vi "Multi_Run_Prog.vi"(0 "Command filename":path, 1 "Setup mode":T9(ring)) -> ()   [LabVIEW 2014]
uses:
  Anemometry Sub Vis/Gen Trav/Traverse_cluster.ctl
  Anemometry Sub Vis/Gen Trav/Spacing.ctl
  Anemometry Sub Vis/Controls/Multi_run_mode.ctl
  Anemometry Sub Vis/Gen Trav/Route mapping/Route_Display_Mode.ctl
  Anemometry Sub Vis/Controls/User_Specific_mode.ctl
  Anemometry Sub Vis/Controls/Multi_Run_Case.ctl
  Anemometry Sub Vis/Gen Trav/Multi_Run_Status.ctl
  Anemometry Sub Vis/Controls/Tunnel_Coordinates.ctl
  Anemometry Sub Vis/Controls/Post_Process.ctl
  ADAM Client/Sub VIs/ADAM Controls/Traverse_Level_State.ctl
  ADAM Client/Sub VIs/ADAM Controls/Tunnel_speed_mode.ctl
  Anemometry Sub Vis/Controls/Overhead.ctl
  ADAM Client/Sub VIs/ADAM Controls/Remember_value_mode.ctl
  Anemometry Sub Vis/Gen Trav/Trav_mode.ctl
  Anemometry Sub Vis/Controls/Home.ctl
  ADAM Client/Sub VIs/ADAM Controls/Client_Source_Status.ctl
  ADAM Client/Sub VIs/ADAM Controls/Update_scan_value.ctl
  Anemometry Sub Vis/File/Setup_Filetype.ctl
  Anemometry Sub Vis/Globals/Meas_global.vi
  Anemometry Sub Vis/Globals/Trav_pos_global.vi
  Anemometry Sub Vis/Globals/Preference_global.vi
  Anemometry Sub Vis/Gen Trav/Route mapping/Route_mapping_global.vi
  ADAM Serial/Instrument drivers/Traverses/~subVIs/DriveConfigGlobal.vi
  Anemometry Sub Vis/Globals/Extra_Commands_Global.vi
panel:
  out "Last Row Run":i32
  in  "Stop after Repeats":bool
  in  "Jump Bad Positions":bool
  in  "Work in Tunnel Coordinates?":T1
  out "Current Overhead Factor":dbl format="%.3f"
  out "Estimated Completion time":string
  out "Max Tunnel Speed":dbl format="%.2f"
  out "Pause message":string
  in  "Pause":bool
  out "Non Starter":bool
  out "No of Rows":i32
  out "Status":T2
  in  "Synchronization Start No":i32=1 min=1 max=100
  out "Multi Run Case":T3
  out "Simulate/Run":T4
  in  "Display Mode":T5=enum."Display View on Crash"
  in  "stop":bool
  out "Currently on Row":i32
  in  "Table":T6[](array[typedef]) {"Row Duration (mins)" format="%#.1f"; "Row No" min=0; "Trace Gas Concentration (%)" min=0.0 format="%#.2f"; "Emission Rate (l/min)" format="%#.2f"; "Tunnel Speed" format="%#.2f"; "Start X" format="%#.2f"; "Start Y" format="%#.2f"; "Start Z" format="%#.2f"; "End X" format="%#.2f"; "End Y" format="%#.2f"; "End Z" format="%#.2f"; "Averaging time (min)" min=0.0 format="%#.2f"}
  # "X           Y            Z"
  # "Start"
  # "End"
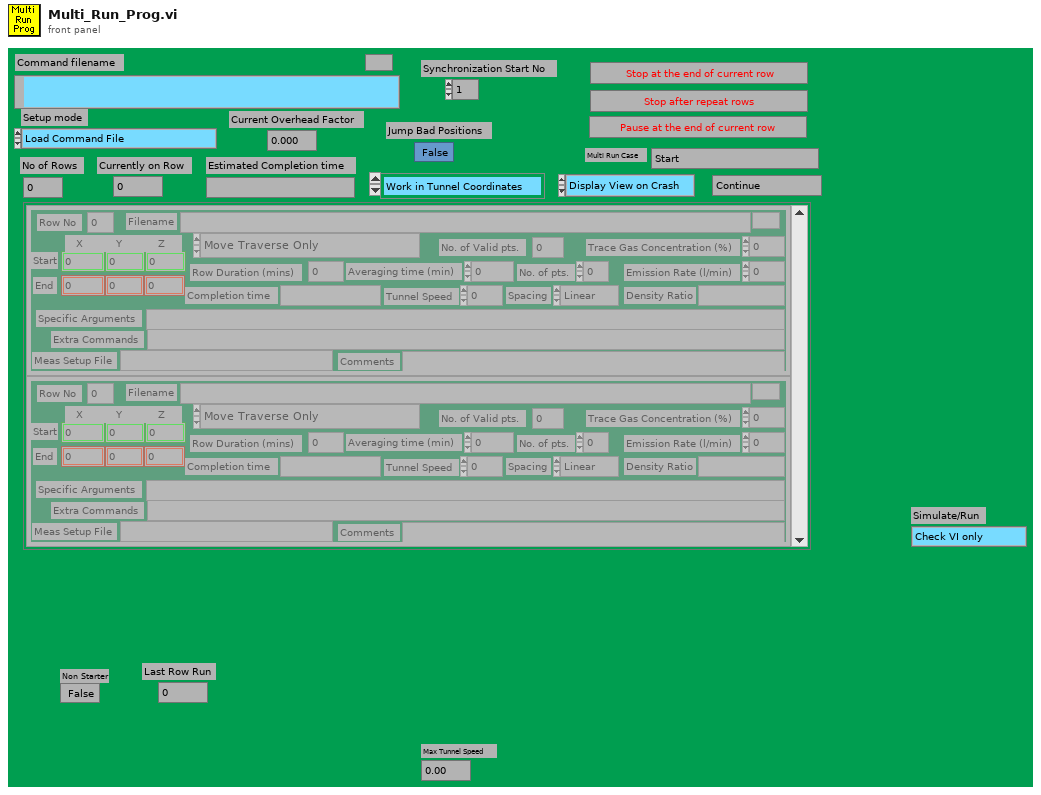
[diagram p1: front panel]
types:
  T1 = typedef "Tunnel_Coordinates.ctl" = enum16{"Work in Tunnel Coordinates", "Work in Model Coordinates"}
  T2 = typedef "Multi_Run_Status.ctl" = enum16{"Continue", "Jump to Next Point", "Jump to Next Row", "Jump To Fall Back", "Terminate Run"}
  T3 = typedef "Multi_Run_Case.ctl" = enum16{"Start", "Load Setup From File", "Has file been edited in Excel?", "Check Max Tunnel Speed", "Pre Check Row", "Check Rows", "Remove blank end rows", "Do results files already exist?", "FFID Bkgnd Measurements?", "First Save Setup file", "Setup Route checking", "Initialise Measurement Prog", "Input Current Position", "Experimental setup control", "Check source flowrates", "Setup for running mode", "Skip Blank Rows", "Which row to execute next", "Evaluate IF Statement", "Perform Measurement Setup", "Set Measurement Conditions", "Execute Row", "Calculate Row TIme", "Update time estimate", "Pause Multi Run Program", "Do Another Row?", "Find Next Fall Back Row", "Shut down source etc", "Email results to users", "Save run efficiency", "Remove Skipped Commands", "Show jumped positions", "Save Setup to File", "End"}
  T4 = typedef "User_Specific_mode.ctl" = enum16{"Check VI only", "Run VI"}
  T5 = typedef "Route_Display_Mode.ctl" = enum16{"Display View Always", "Display View on Crash"}
  T6 = typedef "Traverse_cluster.ctl" = cluster{"Start X":dbl, "Start Y":dbl, "Start Z":dbl, "End X":dbl, "End Y":dbl, "End Z":dbl, "No. of pts.":i32, "Spacing":T7, "Filename":path, "Tunnel Speed":dbl, "Averaging time (min)":dbl, "Extra Commands":string, "Specific Arguments":string, "Emission Rate (l/min)":dbl, "Trace Gas Concentration (%)":dbl, "Density Ratio":string, "Comments":string, "Row No":i32, "Row Type Selector":T8, "Completion time":string, "Row Duration (mins)":dbl, "No. of Valid pts.":i32, "Meas Setup File":string}
  T7 = typedef "Spacing.ctl" = enum16{"Linear", "Log", "Gauss", "Specified", "N/A"}
  T8 = typedef "Multi_run_mode.ctl" = enum16{"Move Traverse Only", "Set Tunnel Speed Only", "Set Source Only", "Set Measurement Conditions", "Single Measurement", "Vertical Profile", "Lateral Profile", "Longitudinal Profile", "Explore Volume", "Multi-Axis Profile", "Auto Calibrate", "Meas Fast FID Bkgnd", "Check Beam Power", "Scanning Valve Measurement", "Run VI Named:", "Set ADAM Ch", "Wait (minutes)", "Send Message", "Synchronize With:", "Fall Back to this Row", "Turn Off Row Repeating", "Blank Row", "Traverse 3D Volume"}
  T9 = enum16{"Load Command File", "Save Command File", "Check Multi Run Prog", "Check Multi Run Prog With Live Moves", "Run Multi Run Prog"}
  T10 = typedef "Post_Process.ctl" = enum16{"Take New Data", "Post Process Raw Data File"}
  T11 = typedef "Traverse_Level_State.ctl" = enum16{"Running", "Complete"}
  T12 = enum32{"existing file", "new file", "new or existing file", "existing dir", "new dir", "new or existing dir", "existing file (use LLBs)", "new file (use LLBs)", "new or existing file (use LLBs)", "new or existing file or directory (use LLBs)"}
  T13 = typedef "Tunnel_speed_mode.ctl" = enum16{"Set Speed", "Set Speed then wait", "Is tunnel speed allowable?"}
  T14 = enum16{"All Channel Names", "Valid Channel Names"}
  T15 = typedef "Overhead.ctl" = enum16{"Update total times", "Read Current Overhead", "Re Scale totals to 3 hrs", "Initialise totals to 3hr"}
  T16 = typedef "Remember_value_mode.ctl" = enum16{"Read only", "Read and Write"}
  T17 = typedef "Home.ctl" = enum16{"Don't Home", "Home  +X", "Home  -X", "Home  +Y", "Home  -Y", "Home  +Z", "Home  -Z"}
  T18 = typedef "Trav_mode.ctl" = enum16{"Move traverse", "Read traverse position", "Teach Position"}
  T19 = typedef "Client_Source_Status.ctl" = enum16{"Not Using", "Using", "Must Have"}
  T20 = typedef "Update_scan_value.ctl" = cluster{"Channel Name":string, "New Value":dbl}
  T21 = typedef "Setup_Filetype.ctl" = enum16{"Measurement Setups", "Calibration Setups", "General", "Results File Plotter Setups", "Speed Calib Tweaks"}
  T22 = typedef "AxisConfigCluster.ctl" = cluster{"Channel Properties":T23, "Static Drive Configuration":T24}
  T23 = typedef "DriveProperties.ctl" = cluster{"Channel Name":string, "Vel. Default":dbl, "Acc. Default":dbl, "Vel. Max":dbl, "Vel. Min":dbl, "Acc. Max":dbl, "Acc. Min":dbl, "Pulses/unit":dbl, "Address":u8, "Pulse Offset":i32, "Pos Tolerance":dbl, "Pulses/rev":dbl, "Backlash/Eng units":dbl, "Current Pos":dbl, "Ch Status":enum16{"Active", "Offline", "Simulate"}, "Port Name":string, "Axis Transform mode":string, "Metadata Ch Name":string, "Type":string}
  T24 = typedef "DriveStaticConfig.ctl" = cluster{"Correction Gain % (CG)":u16, "Dead Band (DB)":i32, "Dead Band Window (DW)":i32, "Encoder Resolution (ER)":i32, "Step Mode  (FSB)":u16, "Position Maintenance (FSC)":u16, "Stop on Stall (FSD)":u16, "Activate OP1 on stall (FSE)":u16, "Stop on Trigger 3 (FSF)":u16, "OP2 in Deadband (FSG)":u16, "Stall Detect (FSH)":u16, "Limit Disable (LD)":u16, "Motor Resolution (MR)":enum16{"200", "400", "1000", "2000", "4000", "5000", "10000", "12800", "18000", "20000", "21600", "25000", "25400", "25600", "36000", "50000", "278528", "425984", "507904", "614400", "655360", "819200", "1024000"}, "Limit Switch Sense (OSA)":u16, "Home Position (OSB)":u16, "Home Switch Sense (OSC)":u16, "Encoder Z for Home (OSD)":u16, "Reference edge of Home (OSH)":u16, "RS232 Echo Control (SSA)":u16, "Buffer at Limit (SSG)":u16, "Buffer at Stop (SSH)":u16, "Indexer Mode  (FSA)":u16, "Type":string, "ConfigString":string, "De Power Motor":enum16{"TRUE", "FALSE"}}
  T25 = typedef "Status_Cluster.ctl" = cluster{"Status":T2, "Error Type":string, "Error Description":string}
  T26 = typedef "Server_Comms.ctl" = enum16{"Server Link Healthy", "Do Not Link To Server"}
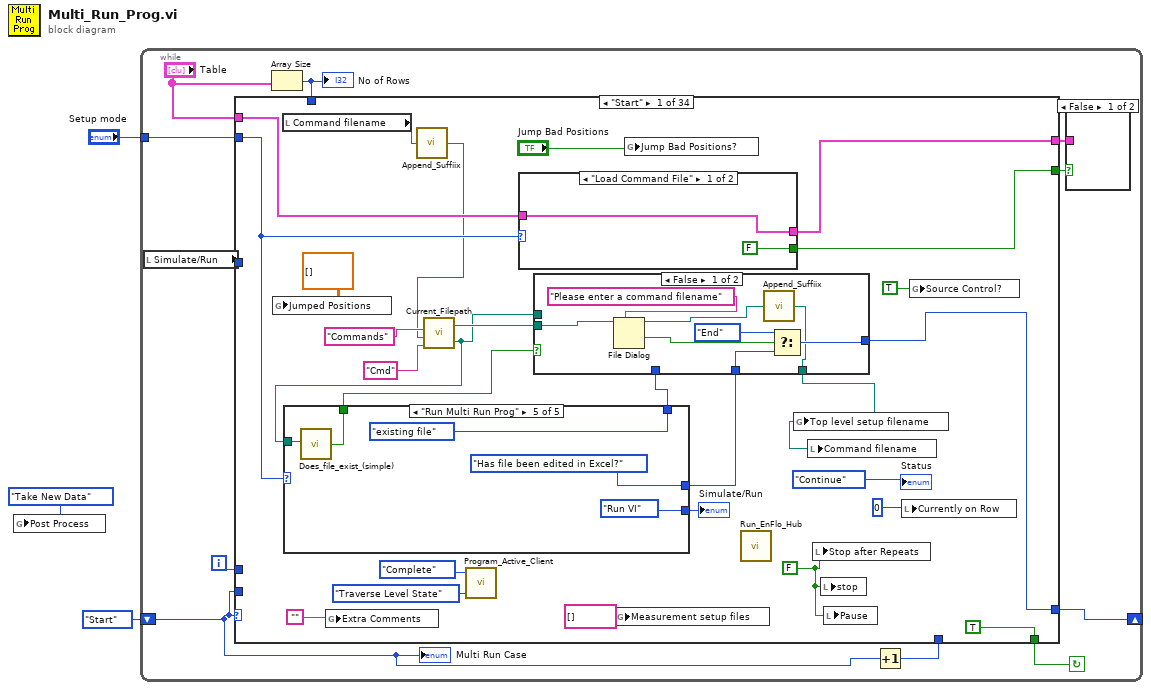
[diagram p0: block diagram]
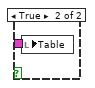
[diagram p2: hidden frame]
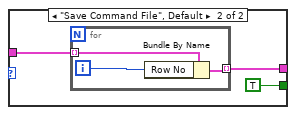
[diagram p3: hidden frame]
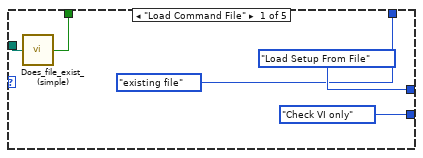
[diagram p5: hidden frame]
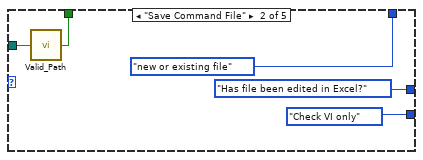
[diagram p6: hidden frame]
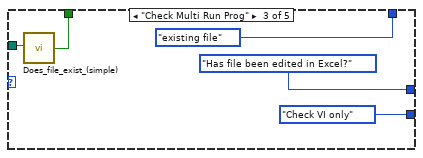
[diagram p7: hidden frame]
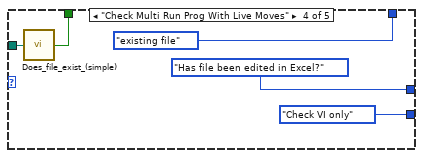
[diagram p8: hidden frame]
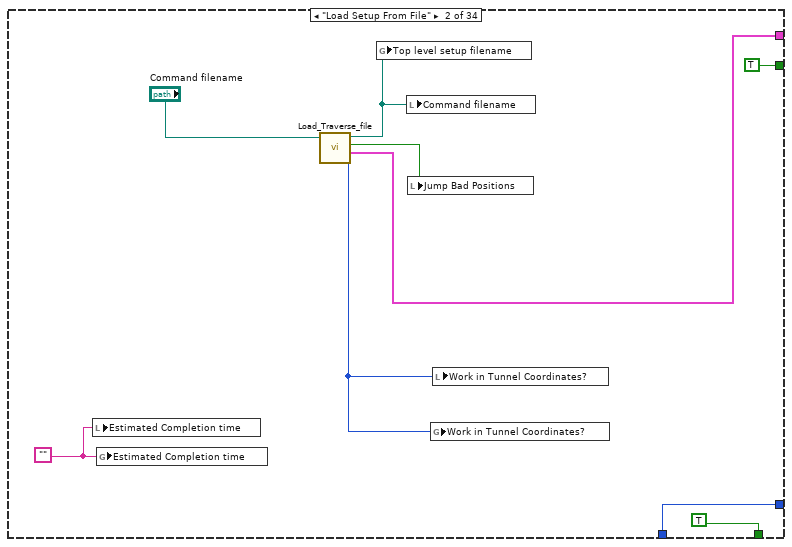
[diagram p9: hidden frame]
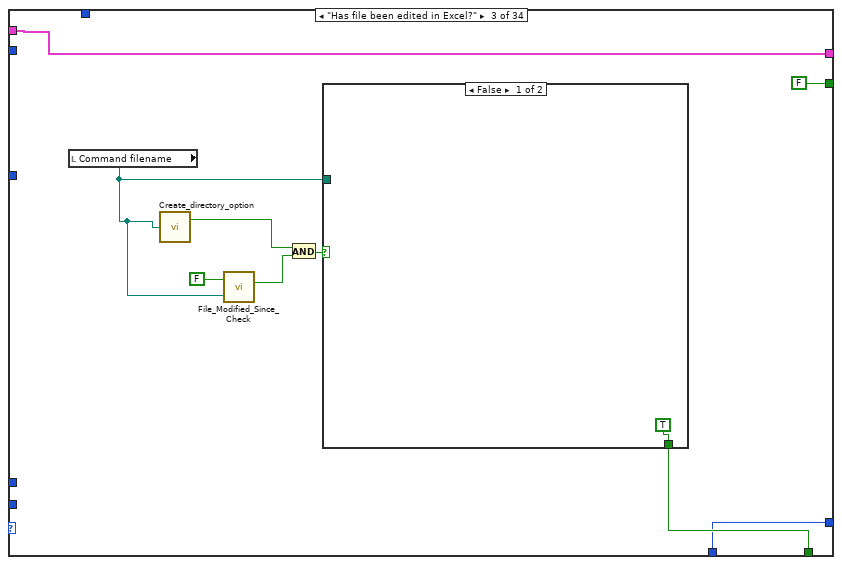
[diagram p10: hidden frame]
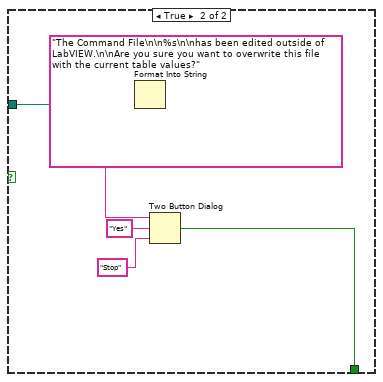
[diagram p11: hidden frame]
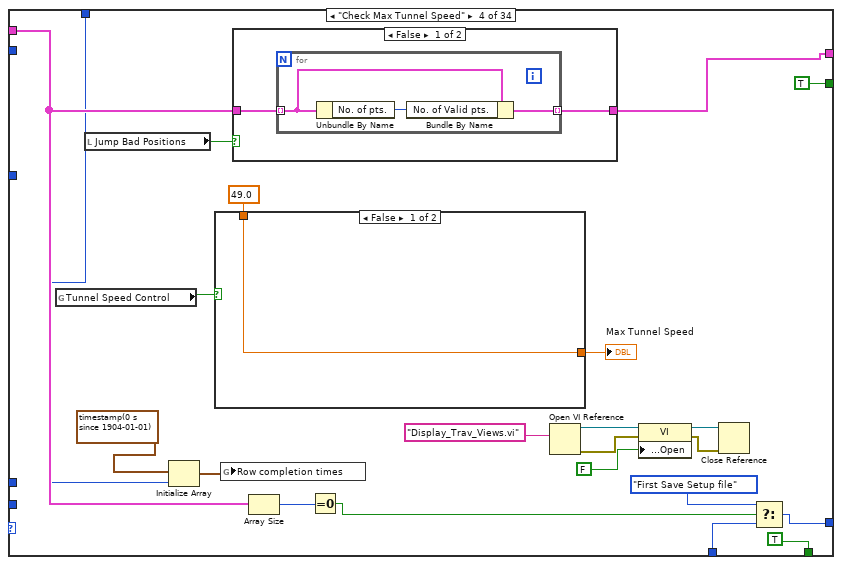
[diagram p12: hidden frame]
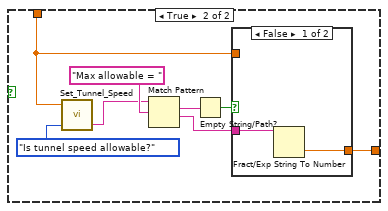
[diagram p14: hidden frame]
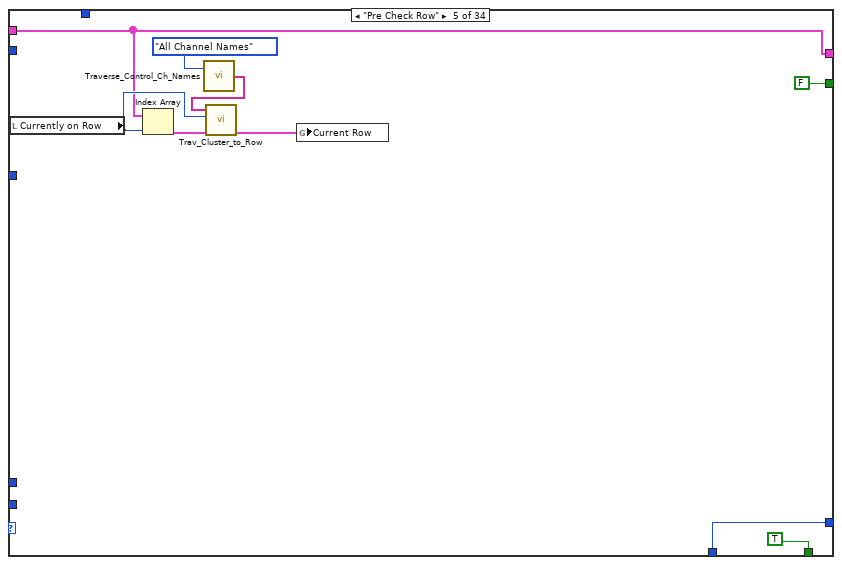
[diagram p16: hidden frame]
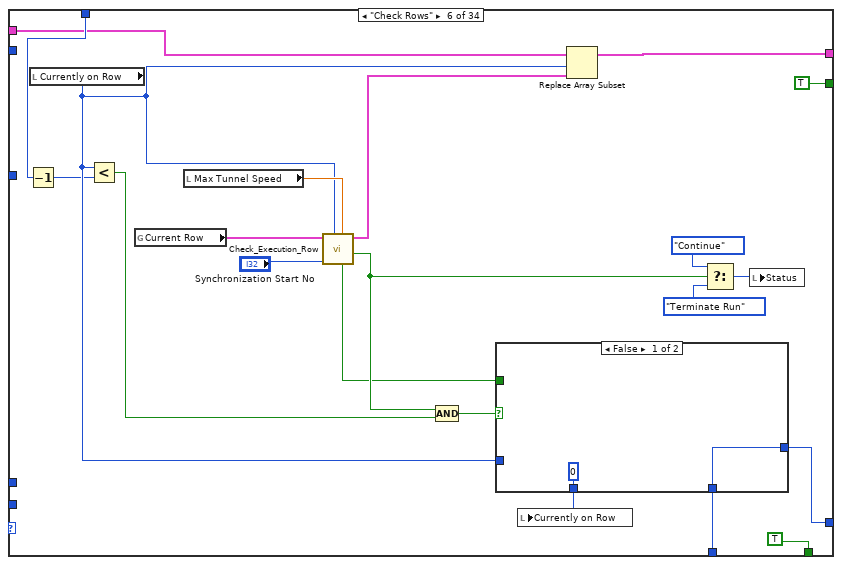
[diagram p17: hidden frame]
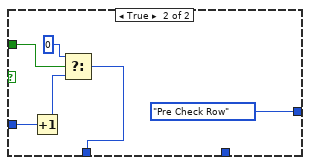
[diagram p18: hidden frame]
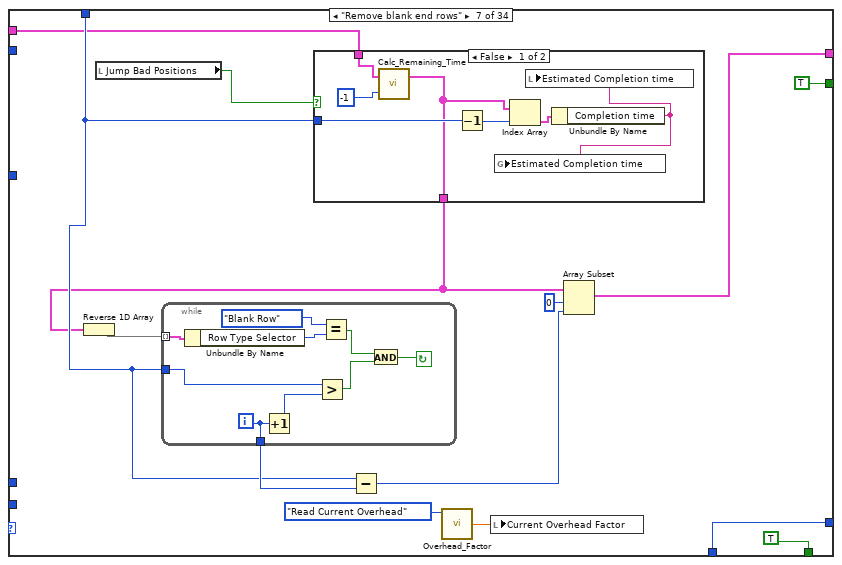
[diagram p19: hidden frame]
diagram:
  n1 = global write "Meas_global.vi" "Post Process"(Post_Process."Take New Data" ("Post Process")) -> ()
  n2 = while {
    shift-left: Multi_Run_Case."Start" ("Multi Run Case") -> [w10]
    shift-right: [w6] -> _
    tunnel: "Setup mode" -> [w13]
    i -> [w11]
    stop <- w14 continue-if-true
    n3 = local read "Simulate/Run"() -> (w7:T4)
    n4 = Array Size(array="Table") -> (size(s)=w5:i32)
    "No of Rows" <- w5
    n5 = Increment(x=w10) -> (x+1=w12:T3)
    n6 = case shown="\"Start\"" w10 {
      tunnel: [TRUE TRUE w98 TRUE TRUE TRUE TRUE TRUE TRUE TRUE TRUE ("Continue?") TRUE ("Continue?") TRUE TRUE TRUE w518 TRUE ("Continue?") TRUE ("Continue?") TRUE TRUE ("Continue?") TRUE TRUE TRUE TRUE TRUE TRUE TRUE TRUE TRUE TRUE TRUE TRUE TRUE FALSE] -> w14
      tunnel: w13 -> [w28 _ _ _ _ _ _ _ _ w406 _ _ _ _ _ _ _ _ _ _ _ _ _ _ _ _ _ _ _ _ _ _ w1268 _]
      tunnel: "Table" -> [w40 _ w95 w125 w153 w165 w190 w221 w379 w408 w430 w484 w489 w495 w505 w521 w596 w640 w756 w807 w819 w912 w948 w980 w1023 w1069 w1117 w1145 w1165 w1212 w1217 w1226 w1289 w1353]
      tunnel: w7 -> [_ _ _ _ _ _ _ w220 _ _ _ _ _ w499 w504 w520 _ w638 w753 w804 w817 w911 w946 w977 _ w1078 _ _ _ _ _ _ w1279 _]
      tunnel: w10 -> [_ _ _ _ _ _ _ _ _ _ _ _ _ _ _ _ _ _ _ _ _ _ _ _ _ _ _ _ _ _ _ _ _ _]
      tunnel: w12 -> [_ w91 w97 w123 w157 w167 w201 w225 w374 w405 w434 w482 w490 w494 w510 w523 w598 w636 w761 w808 w826 w909 w938 w982 w1026 _ _ w1131 w1167 w1214 w1220 w1234 w1287 w1352]
      tunnel: w11 -> [_ _ _ _ _ _ _ _ _ _ _ _ _ _ _ _ _ _ _ _ _ _ _ _ w1024 _ _ _ _ _ _ _ _ _]
      tunnel: [w38 w91 w97 w122 w157 w166 w201 w225 w374 w401 w434 w481 w490 w494 w507 w523 w598 w637 w760 w808 w827 w909 w938 w982 w1027 w1061 w1114 w1140 w1167 w1214 w1220 w1234 w1287 w1352] -> w6
      tunnel: [w27 TRUE FALSE ("Rows Added ?") TRUE ("Rows Added ?") FALSE TRUE TRUE FALSE FALSE TRUE FALSE FALSE FALSE FALSE FALSE TRUE FALSE ("Rows Added ?") FALSE ("Rows Added ?") FALSE FALSE ("Rows Added ?") FALSE FALSE FALSE TRUE ("Rows Added ?") FALSE FALSE FALSE FALSE FALSE FALSE TRUE TRUE TRUE FALSE] -> w8
      tunnel: w5 -> [_ _ _ w117 _ w171 w192 _ _ _ _ _ _ _ _ _ w599 w639 _ _ _ _ _ w976 _ w1064 _ _ _ _ _ _ _ _]
      tunnel: [w39 w92 w95 w127 w153 w174 w196 w221 w379 w409 w430 w484 w489 w495 w505 w519 w596 w641 w756 w807 w819 w912 w948 w979 w1023 w1069 w1117 w1145 w1165 w1212 w1216 w1226 w1288 w1353] -> w4
      frame "Start" {
        w25 = FALSE ("Measurment setup Found?")
        n7 = global write "Trav_pos_global.vi" "Jumped Positions"(dbl[][] [] ("Jumped Positions")) -> ()
        n8 = local read "Command filename"() -> (w30:path)
        n9 = global write "Meas_global.vi" "Extra Comments"("") -> ()
        n10 = call "Append_Suffiix.vi"("Results file"=w30) -> ("appended path"=w20:path)
        n11 = call "Current_Filepath.vi"("Short_Name"="Cmd" ("Data Type"), "Filename in"=w20, "Data Type"="Commands") -> ("Filename Out"=w17:path, "Directory"=w19:path)  [unwired: 1 in]
        n12 = case shown="\"Run Multi Run Prog\"" w28 {
          tunnel: [User_Specific_mode."Check VI only" ("Simulate/Run") User_Specific_mode."Check VI only" ("Simulate/Run") User_Specific_mode."Check VI only" ("Simulate/Run") User_Specific_mode."Check VI only" ("Simulate/Run") User_Specific_mode."Run VI" ("Simulate/Run")] -> w41
          tunnel: [Multi_Run_Case."Load Setup From File" ("Multi Run Case") Multi_Run_Case."Has file been edited in Excel?" ("Multi Run Case") Multi_Run_Case."Has file been edited in Excel?" ("Multi Run Case") Multi_Run_Case."Has file been edited in Excel?" ("Multi Run Case") Multi_Run_Case."Has file been edited in Excel?" ("Multi Run Case")] -> w37
          tunnel: [T12."existing file" ("select mode (2)") T12."new or existing file" ("select mode (2)") T12."existing file" ("select mode (2)") T12."existing file" ("select mode (2)") T12."existing file" ("select mode (2)")] -> w26
          tunnel: w17 -> [w62 w67 w71 w77 w82]
          tunnel: [w61 w66 w72 w76 w81] -> w16
          frame "Load Command File" {
            n13 = call "Does_file_exist_(simple).vi"("Pathname"=w62) -> ("exists?"=w61:bool)
          }
          frame "Save Command File" {
            n14 = call "Valid_Path.vi"("Filename"=w67) -> ("Valid Path?"=w66:bool)
          }
          frame "Check Multi Run Prog" {
            n15 = call "Does_file_exist_(simple).vi"("Pathname"=w71) -> ("exists?"=w72:bool)
          }
          frame "Check Multi Run Prog With Live Moves" {
            n16 = call "Does_file_exist_(simple).vi"("Pathname"=w77) -> ("exists?"=w76:bool)
          }
          frame "Run Multi Run Prog" {
            n17 = call "Does_file_exist_(simple).vi"("Pathname"=w82) -> ("exists?"=w81:bool)
          }
        }
        "Simulate/Run" <- w41
        n18 = call "Program_Active_Client.vi"("Mode"=enum16{"Program Active", "Traverse Level State"}."Traverse Level State", "Traverse level State"=Traverse_Level_State."Complete") -> ()  [unwired: 1 in, 3 out]
        n19 = case shown="\"Load Command File\"" w28 {
          tunnel: w40 -> [w44 w47]
          tunnel: [w44 w46] -> w39
          tunnel: [FALSE TRUE] -> w27
          frame "Load Command File" {
          }
          frame "Save Command File", Default {
            n20 = for {
              tunnel: w47 -> [w50] mode=indexing
              tunnel: [w49] -> w46 mode=indexing
              i -> [w48]
              n21 = Bundle By Name(cluster=w50, "Row No"=w48) -> (w49:T6)
            }
          }
        }
        n22 = case shown="False" w16 {
          tunnel: [w56 w60] -> w38
          tunnel: w37 -> [w57 w60]
          tunnel: w17 -> [_ w59]
          tunnel: [w55 w59] -> w29
          tunnel: w26 -> [_ _]
          tunnel: w19 -> [w51 _]
          frame False {
            n23 = File Dialog(7:"Please enter a command filename" ("prompt"), 11:w51) -> (1:w53:bool, 3:w54:path)  [unwired: 1 in, 6 out]
            n24 = call "Append_Suffiix.vi"("Results file"=w54) -> ("appended path"=w55:path)
            n25 = Select(t=Multi_Run_Case."End" ("Multi Run Case"), s=w53, f=w57) -> (s? t:f=w56:T3)
          }
          frame True {
          }
        }
        n26 = global write "Trav_pos_global.vi" "Measurement setup files"(string[] [] ("Measurement setup files")) -> ()
        n27 = global write "Trav_pos_global.vi" "Jump Bad Positions?"("Jump Bad Positions") -> ()
        n28 = call "Run_EnFlo_Hub.vi"() -> ()  [unwired: 8 out]
        n29 = global write "Trav_pos_global.vi" "Top level setup filename"(w29) -> ()
        n30 = local write "Command filename"(w29) -> ()
        n31 = local write "Stop after Repeats"(w25) -> ()
        n32 = local write "stop"(w25) -> ()
        n33 = local write "Pause"(w25) -> ()
        n34 = local write "Currently on Row"(0 ("Currently on Row")) -> ()
        n35 = global write "Trav_pos_global.vi" "Source Control?"(TRUE ("Source Control?")) -> ()
        "Status" <- Multi_Run_Status."Continue" ("Status")
      }
      frame "Load Setup From File" {
        w87 = ""
        n36 = local write "Estimated Completion time"(w87) -> ()
        n37 = global write "Trav_pos_global.vi" "Estimated Completion time"(w87) -> ()
        n38 = call "Load_Traverse_file.vi"("Setup filename"="Command filename") -> ("Setup filename Out"=w89:path, "Jump Bad Positions"=w86:bool, "Table"=w92:T6[], "Work in Tunnel Coordinates?"=w88:T1)  [unwired: 2 out]
        n39 = global write "Trav_pos_global.vi" "Top level setup filename"(w89) -> ()
        n40 = local write "Command filename"(w89) -> ()
        n41 = local write "Jump Bad Positions"(w86) -> ()
        n42 = global write "Trav_pos_global.vi" "Work in Tunnel Coordinates?"(w88) -> ()
        n43 = local write "Work in Tunnel Coordinates?"(w88) -> ()
      }
      frame "Has file been edited in Excel?" {
        n44 = local read "Command filename"() -> (w99:path)
        n45 = call "Create_directory_option.vi"("Filename"=w99) -> ("Path is to existing File"=w102:bool)  [unwired: 1 out]
        n46 = call "File_Modified_Since_Check.vi"("Pathname"=w99, "Just Modified?"=FALSE) -> ("Modified?"=w101:bool)
        n47 = And(x=w102, y=w101) -> (x .and. y?=w103:bool)
        n48 = case shown="False" w103 {
          tunnel: w99 -> [_ w110]
          tunnel: [TRUE ("T button?") w105] -> w98
          frame False {
          }
          frame True {
            n49 = Format Into String(format string="The Command File\n\n%s\n\nhas been edited outside of LabVIEW.\n\nAre you sure you want to overwrite this file  with the current table values?" ("Format String"), w110) -> (resulting string=w108:string)  [unwired: 2 in, 1 out]
            n50 = Two Button Dialog(message=w108, 1:"Stop" ("F button name (\"Cancel\")"), 2:"Yes" ("T button name (\"OK\")")) -> (T button?=w105:bool)
          }
        }
      }
      frame "Check Max Tunnel Speed" {
        n51 = global read "Preference_global.vi" "Tunnel Speed Control"() -> (w128:bool)
        n52 = local read "Jump Bad Positions"() -> (w126:bool)
        n53 = Initialize Array(timestamp(0 s since 1904-01-01) ("seconds since 1Jan1904"), w117) -> (w118:timestamp[])
        n54 = case shown="False" w128 {
          tunnel: 49.0 ("Tunnel Velocity m/s") -> [w139 w140]
          tunnel: [w139 w142] -> w130
          frame False {
          }
          frame True {
            n55 = call "Set_Tunnel_Speed.vi"("Mode"=Tunnel_speed_mode."Is tunnel speed allowable?", "Tunnel Velocity m/s"=w140) -> ("Error String"=w145:string)  [unwired: 1 in, 2 out]
            n56 = Match Pattern(string=w145, regular expression="Max allowable = ") -> (match substring=w144:string, after substring=w141:string)  [unwired: 3 out]
            n57 = Empty String/Path?(string/path=w144) -> (empty?=w143:bool)
            n58 = case shown="False" w143 {
              tunnel: [w148 w150] -> w142
              tunnel: w140 -> [_ w150]
              tunnel: w141 -> [w149 _]
              frame False {
                n59 = Fract/Exp String To Number(string=w149) -> (number=w148:dbl)  [unwired: 4 out]
              }
              frame True {
              }
            }
          }
        }
        "Max Tunnel Speed" <- w130
        n60 = global write "Trav_pos_global.vi" "Row completion times"(w118) -> ()
        n61 = case shown="False" w126 {
          tunnel: w125 -> [w134 w138]
          tunnel: [w133 w138] -> w127
          frame False {
            n62 = for {
              tunnel: w134 -> [w136] mode=indexing
              tunnel: [w135] -> w133 mode=indexing
              n63 = Unbundle By Name(w136) -> ("No. of pts."=w137:i32)
              n64 = Bundle By Name(cluster=w136, "No. of Valid pts."=w137) -> (w135:T6)
            }
          }
          frame True {
          }
        }
        n65 = Array Size(array=w125) -> (size(s)=w124:i32)
        n66 = Equal To 0?(x=w124) -> (x = 0?=w121:bool)
        n67 = Open VI Reference(vi path="Display_Trav_Views.vi" ("VI path")) -> (vi reference=w116:refnum<vi>, error out=w115:errorcluster)  [unwired: 1 in, 4 out]
        n68 = property class="VI"(reference=w116, error in=w115, "Front Panel Window:Open"=FALSE) -> (reference out=w113:refnum<vi>, error out=w112:errorcluster)
        n69 = Close Reference(reference=w113, error in (no error)=w112) -> ()  [unwired: 1 out]
        n70 = Select(t=Multi_Run_Case."First Save Setup file" ("Multi Run Case"), s=w121, f=w123) -> (s? t:f=w122:T3)
      }
      frame "Pre Check Row" {
        n71 = local read "Currently on Row"() -> (w154:i32)
        n72 = Index Array(array=w153, index=w154) -> (element=w155:T6)
        n73 = call "Traverse_Control_Ch_Names.vi"("Mode"=T14."All Channel Names") -> ("Channel names"=w151:string[])  [unwired: 1 in]
        n74 = call "Trav_Cluster_to_Row.vi"("Traverse line in"=w155, "Row Number"=w154, "Channel names"=w151) -> ("Traverse line Out"=w156:T6)  [unwired: 4 out]
        n75 = global write "Trav_pos_global.vi" "Current Row"(w156) -> ()
      }
      frame "Check Rows" {
        n76 = Decrement(x=w171) -> (x-1=w162:i32)
        n77 = local read "Currently on Row"() -> (w163:i32)
        n78 = Less?(x=w163, y=w162) -> (x < y?=w170:bool)
        n79 = global read "Trav_pos_global.vi" "Current Row"() -> (w160:T6)
        n80 = local read "Max Tunnel Speed"() -> (w173:dbl)
        n81 = call "Check_Execution_Row.vi"("Execution Row"=w160, "Synchronization Start No"="Synchronization Start No", "Row Index"=w163, "Max Tunnel Speed"=w173) -> ("Editted Row"=w161:bool, "Execution Row Out"=w164:T6, "Continue?"=w172:bool)  [unwired: 1 in, 3 out]
        n82 = Compound Arithmetic op=AND(w172, w170) -> (w169:bool)
        n83 = case shown="False" w169 {
          tunnel: [0 w184] -> w168
          tunnel: w163 -> [_ w188]
          tunnel: w167 -> [w182 _]
          tunnel: [w182 Multi_Run_Case."Pre Check Row" ("Multi Run Case")] -> w166
          tunnel: w161 -> [_ w186]
          frame False {
          }
          frame True {
            n84 = Increment(x=w188) -> (x+1=w185:i32)
            n85 = Select(t=0, s=w186, f=w185) -> (s? t:f=w184:i32)
          }
        }
        n86 = local write "Currently on Row"(w168) -> ()
        n87 = Replace Array Subset(array=w165, new element=w164, index=w163) -> (w174:T6[])
        n88 = Select(t=Multi_Run_Status."Continue" ("Status"), s=w172, f=Multi_Run_Status."Terminate Run" ("Status")) -> (s? t:f=w178:T2)
        n89 = local write "Status"(w178) -> ()
      }
      frame "Remove blank end rows" {
        n90 = local read "Jump Bad Positions"() -> (w189:bool)
        n91 = case shown="False" w189 {
          tunnel: w192 -> [w207 _]
          tunnel: w190 -> [w206 w210]
          tunnel: [w204 w210] -> w191
          frame False {
            n92 = call "Calc_Remaining_Time.vi"("Currently on Row"=-1 ("Start Index"), "Table In"=w206) -> ("Table Out"=w204:T6[])  [unwired: 1 out]
            n93 = Decrement(x=w207) -> (x-1=w209:i32)
            n94 = Index Array(array=w204, index=w209) -> (element=w208:T6)
            n95 = Unbundle By Name(w208) -> ("Completion time"=w203:string)
            n96 = global write "Trav_pos_global.vi" "Estimated Completion time"(w203) -> ()
            n97 = local write "Estimated Completion time"(w203) -> ()
          }
          frame True {
          }
        }
        n98 = Reverse 1D Array(array=w191) -> (reversed array=w200:T6[])
        n99 = while {
          tunnel: [w211] -> w198
          tunnel: w192 -> [w215]
          tunnel: w200 -> [w219] mode=indexing
          i -> [w211]
          stop <- w212 continue-if-true
          n100 = Unbundle By Name(w219) -> ("Row Type Selector"=w217:T8)
          n101 = Increment(x=w211) -> (x+1=w216:i32)
          n102 = Greater?(x=w215, y=w216) -> (0:w214:bool)
          n103 = Equal?(x=Multi_run_mode."Blank Row" ("Row Type Selector"), y=w217) -> (x = y?=w213:bool)
          n104 = And(x=w213, y=w214) -> (x .and. y?=w212:bool)
        }
        n105 = Subtract(x=w192, y=w198) -> (x-y=w197:i32)
        n106 = call "Overhead_Factor.vi"("Mode"=Overhead."Read Current Overhead") -> ("Current Overhead Factor"=w193:dbl)  [unwired: 3 in]
        n107 = local write "Current Overhead Factor"(w193) -> ()
        n108 = Array Subset(array=w191, index=0 ("Array Index"), length=w197) -> (w196:T6[])
      }
      frame "Do results files already exist?" {
        n109 = for {
          tunnel: w221 -> [w237] mode=indexing
          tunnel: [w235] -> w227 mode=indexing
          shift-right: [w231] -> _
          shift-left: path[] [] -> [w232]
          tunnel: w220 -> [w229]
          n110 = Unbundle By Name(w237) -> ("Specific Arguments"=w228:string, "Emission Rate (l/min)"=w236:dbl, "Row Type Selector"=w234:T8, "Filename"=w233:path)
          n111 = while {
            shift-left: w232 -> [w245]
            shift-right: [w244] -> w231
            tunnel: w233 -> [w246]
            tunnel: w234 -> [w250]
            shift-left: 0 -> [w251]
            shift-right: [w247] -> _
            tunnel: w229 -> [w241]
            shift-right: [w240] -> _
            shift-left: _ -> [w239]
            tunnel: w228 -> [w238]
            stop <- w249 continue-if-true
            n112 = Increment(x=w251) -> (x+1=w248:i32)
            n113 = case shown="0, Default" w251 {
              tunnel: w250 -> [w260 _ _ _ _ _ _ _ _ _ _ _]
              tunnel: [w255 w280 w285 w292 w297 TRUE ("exists?") TRUE ("exists?") FALSE ("exists?") FALSE ("exists?") TRUE ("true") w354 w367] -> w249
              tunnel: w248 -> [w262 w283 w288 w291 w298 w303 w314 w325 w336 w340 w352 _]
              tunnel: [w262 w283 w288 w291 w298 w301 w313 w325 w336 w341 w352 w366] -> w247
              tunnel: [w261 w282 w287 w290 w295 w311 w322 w327 w329 w338 w356 w372] -> w244
              tunnel: w245 -> [w261 w282 w287 w290 w296 w311 w322 w327 w329 w338 w356 w372]
              tunnel: w246 -> [w254 _ _ _ _ _ _ _ _ _ _ _]
              tunnel: 7 -> [_ _ _ _ _ _ _ _ _ w339 _ w366]
              tunnel: 9 -> [_ _ _ _ _ w302 _ _ _ _ _ _]
              tunnel: w241 -> [_ _ _ _ _ _ _ _ _ _ w355 _]
              tunnel: [w253 w279 w284 w289 w294 w299 w312 w323 w328 w337 w353 w365] -> w240
              tunnel: w239 -> [_ w279 w284 w289 w294 w299 w312 w323 w328 w337 w353 w365]
              tunnel: w238 -> [w252 _ _ _ _ _ _ _ _ _ _ _]
              frame 0, Default {
                n114 = case shown="\"Send Message\"" w260 {
                  tunnel: [TRUE w270 FALSE FALSE] -> w257
                  tunnel: w254 -> [w263 w269 w275 w277]
                  tunnel: w252 -> [_ w267 _ _]
                  tunnel: [w263 w269 w275 w277] -> w253
                  frame "Move Traverse Only", Default {
                  }
                  frame "Run VI Named:" {
                    n115 = Match Pattern(string=w267, regular expression=";") -> (before substring=w266:string)  [unwired: 4 out]
                    n116 = call <vilib>:"Trim Whitespace.vi"("string"=w266) -> ("trimmed string"=w265:string)  [unwired: 1 in]
                    n117 = Equal?(x=w265, y="Pressure_Tapped_Cube.vi") -> (x = y?=w271:bool)
                    n118 = Equal?(x=w265, y="Take_Data_on_the_Move.vi") -> (x = y?=w272:bool)
                    n119 = Or(x=w271, y=w272) -> (x .or. y?=w270:bool)
                  }
                  frame "Auto Calibrate" {
                  }
                  frame "Send Message" {
                  }
                }
                n120 = local read "Status"() -> (w258:T2)
                n121 = Not Equal?(x=Multi_Run_Status."Terminate Run" ("Status"), y=w258) -> (x != y?=w256:bool)
                n122 = And(x=w257, y=w256) -> (x .and. y?=w255:bool)
              }
              frame 1 {
                n123 = Not Equal?(x=path "", y=w279) -> (x != y?=w280:bool)
              }
              frame 2 {
                n124 = Not Equal?(x=w284, y=path "") -> (x != y?=w285:bool)
              }
              frame 3 {
                n125 = Search 1D Array(1D array=w290, element=w289) -> (index of element=w293:i32)  [unwired: 1 out]
                n126 = Less Than 0?(x=w293) -> (x < 0?=w292:bool)
              }
              frame 4 {
                n127 = Build Array (concatenate)(w296, w294) -> (w295:path[])
                n128 = call "Does_file_exist_(simple).vi"("Pathname"=w294) -> ("exists?"=w297:bool)
              }
              frame 5 {
                n129 = Path To String(path=w299) -> (string=w310:string)
                n130 = global read "Meas_global.vi" "Start Time of experiment"() -> (w305:dbl)
                n131 = Concatenate Strings(w310, "Append" ("Substring")) -> (w308:string)
                n132 = call "Remember_value.vi"("Mode"=Remember_value_mode."Read only", "Ch name"=w308) -> ("Output Value"=w306:dbl)  [unwired: 1 in]
                n133 = Not Equal?(x=w305, y=w306) -> (x != y?=w304:bool)
                n134 = Select(t=w303, s=w304, f=w302) -> (s? t:f=w301:i32)
              }
              frame 6 {
                n135 = Increment(x=w314) -> (x+1=w315:i32)
                n136 = Format Into String(format string="The results filename \"%s\" already exists.\nDo you wish to append to this file during the run?" ("Format String"), w312) -> (resulting string=w319:string)  [unwired: 2 in, 1 out]
                n137 = Two Button Dialog(message=w319, 1:"Abort Run" ("F button name (\"Cancel\")"), 2:"Append" ("T button name (\"OK\")")) -> (T button?=w316:bool)
                n138 = Select(t=w315, s=w316, f=w314) -> (s? t:f=w313:i32)
              }
              frame 7 {
                n139 = local write "Status"(Multi_Run_Status."Terminate Run" ("Status")) -> ()
              }
              frame 8 {
                n140 = Path To String(path=w328) -> (string=w335:string)
                n141 = Concatenate Strings(w335, "Append" ("Substring")) -> (w333:string)
                n142 = global read "Meas_global.vi" "Start Time of experiment"() -> (w330:dbl)
                n143 = call "Remember_value.vi"("Mode"=Remember_value_mode."Read and Write", "Input Value"=w330, "Ch name"=w333) -> ()  [unwired: 1 out]
              }
              frame 9 {
                n144 = call "Read_File_Simple.vi"("Filename"=w337) -> ("string"=w344:string)  [unwired: 2 in, 7 out]
                n145 = call "Is_it_a_Results_File.vi"("character string"=w344) -> ("Results File?"=w343:bool)  [unwired: 2 out]
                n146 = case shown="True" w343 {
                  tunnel: w337 -> [w347 _]
                  tunnel: [w345 w351] -> w341
                  tunnel: w340 -> [_ w351]
                  tunnel: w339 -> [w345 _]
                  frame False {
                    n147 = Path To String(path=w347) -> (string=w349:string)
                    n148 = Format Into String(format string="The File %s is not in the correct Results file format.\nCheck that it is tab delimited rather than excel format, or choose another file." ("Format String"), w349) -> (resulting string=w346:string)  [unwired: 2 in, 1 out]
                    n149 = One Button Dialog(message=w346, button name ("OK")="Stop") -> ()  [unwired: 1 out]
                  }
                  frame True {
                  }
                }
              }
              frame 10 {
                n150 = case shown="\"Check VI only\", Default" w355 {
                  tunnel: w353 -> [_ w364]
                  tunnel: [FALSE ("exists?") w358] -> w354
                  frame "Check VI only", Default {
                  }
                  frame "Run VI" {
                    n151 = call "Open_File_for_write.vi"("append to file? (new file:F)"=TRUE, "file path"=w364) -> ("error out"=w362:errorcluster, "refnum"=w363:refnum<file>)  [unwired: 1 in, 7 out]
                    n152 = Unbundle By Name(w362) -> ("code"=w361:i32)
                    n153 = Close File(refnum=w363, error in=w362) -> ()  [unwired: 2 out]
                    n154 = Equal?(x=10 ("code"), y=w361) -> (x = y?=w358:bool)
                  }
                }
              }
              frame 11 {
                n155 = Path To String(path=w365) -> (string=w370:string)
                n156 = Format Into String(format string="The File %s is already open in another application." ("Format String"), w370) -> (resulting string=w369:string)  [unwired: 2 in, 1 out]
                n157 = One Button Dialog(message=w369, button name ("OK")="Stop") -> (true=w367:bool)
              }
            }
          }
          n158 = Greater Than 0?(x=w236) -> (x > 0?=w235:bool)
        }
        n159 = Or Array Elements(Boolean array=w227) -> (logical OR=w223:bool)
        n160 = global write "Trav_pos_global.vi" "Source Control?"(w223) -> ()
      }
      frame "FFID Bkgnd Measurements?" {
        n161 = for {
          tunnel: w379 -> [w395] mode=indexing
          tunnel: [w383] -> w378 mode=indexing
          tunnel: [w384] -> w377 mode=indexing
          n162 = Unbundle By Name(w395) -> ("Row Type Selector"=w389:T8, "Specific Arguments"=w391:string)
          n163 = call "Get_array_values_fr_String.vi"("String Value"=w391) -> ("String array"=w392:string[])  [unwired: 1 out]
          n164 = Index Array(array=w392, index=0 ("Index")) -> (element=w388:string)
          n165 = Equal?(x=Multi_run_mode."Auto Calibrate" ("Row Type Selector"), y=w389) -> (x = y?=w385:bool)
          n166 = Equal?(x=w388, y="Concentration") -> (x = y?=w386:bool)
          n167 = Equal?(x=Multi_run_mode."Meas Fast FID Bkgnd" ("Row Type Selector"), y=w389) -> (x = y?=w383:bool)
          n168 = And(x=w385, y=w386) -> (x .and. y?=w384:bool)
        }
        n169 = Or Array Elements(Boolean array=w378) -> (logical OR=w375:bool)
        n170 = Or Array Elements(Boolean array=w377) -> (logical OR=w376:bool)
        n171 = Compound Arithmetic op=AND(invert w375, w376) -> (w373:bool)
        n172 = case shown="True" w373 {
          frame False {
          }
          frame True {
            n173 = One Button Dialog(message="This run automatically calibrates the Fast FID but does not have a Meas Fast FID Bkgnd row" ("format string")) -> ()  [unwired: 2 out]
          }
        }
      }
      frame "First Save Setup file" {
        w396 = -1 ("Currently on Row")
        n174 = case shown="\"Check Multi Run Prog\"" w406 {
          tunnel: [w413 w415 w417 Multi_Run_Case."End" ("Multi Run Case") Multi_Run_Case."End" ("Multi Run Case")] -> w400
          tunnel: w405 -> [w413 w415 w417 _ _]
          tunnel: [w414 w416 w418 w419 w421] -> w399
          frame "Run Multi Run Prog" {
            w414 = FALSE  # Live Traverse Preview?
          }
          frame "Check Multi Run Prog With Live Moves" {
            w416 = TRUE  # Live Traverse Preview?
          }
          frame "Check Multi Run Prog" {
            w418 = FALSE  # Live Traverse Preview?
          }
          frame "Load Command File" {
            w419 = FALSE  # Live Traverse Preview?
          }
          frame "Save Command File" {
            w421 = FALSE  # Live Traverse Preview?
          }
        }
        n175 = local read "Command filename"() -> (w407:path)
        n176 = global write "Trav_pos_global.vi" "Work in Tunnel Coordinates?"("Work in Tunnel Coordinates?") -> ()
        n177 = local write "Currently on Row"(w396) -> ()
        n178 = local write "Last Row Run"(w396) -> ()
        n179 = local read "Jump Bad Positions"() -> (w397:bool)
        n180 = call "Save_Trav_setup.vi"("Work in Tunnel Coordinates?"="Work in Tunnel Coordinates?", "Trav Table"=w408, "Jump Bad Positions"=w397, "Setup filename"=w407) -> ("Trav Table Out"=w409:T6[])  [unwired: 1 out]
        n181 = global write "Meas_global.vi" "Extra Comments"("") -> ()
        n182 = global write "Trav_pos_global.vi" "Live Traverse Preview?"(w399) -> ()
        n183 = local read "Status"() -> (w402:T2)
        n184 = case shown="\"Continue\"" w402 {
          tunnel: [w411 Multi_Run_Case."End" ("Multi Run Case")] -> w401
          tunnel: w400 -> [w411 _]
          frame "Continue" {
          }
          frame "Jump to Next Point", Default {
          }
        }
      }
      frame "Setup Route checking" {
        w426 = string[] []
        n185 = global read "Trav_pos_global.vi" "Work in Tunnel Coordinates?"() -> (w427:T1)
        n186 = for {
          tunnel: w430 -> [w471] mode=indexing
          shift-right: [w462] -> w428
          shift-left: string[] [] -> [w463]
          n187 = Unbundle By Name(w471) -> ("Extra Commands"=w464:string, "Start X"=w468:dbl, "Start Y"=w467:dbl, "Start Z"=w466:dbl)
          n188 = Build Array(w468, w467, w466) -> (w469:dbl[])
          n189 = Not A Number/Path/Refnum?(number/path/refnum=w469) -> (NaN/Path/Refnum?=w470:bool[])
          n190 = Or Array Elements(Boolean array=w470) -> (logical OR=w465:bool)
          n191 = case shown="False" w465 {
            tunnel: w464 -> [w475 _]
            tunnel: w463 -> [w474 w476]
            tunnel: [w473 w476] -> w462
            frame False {
              n192 = call "Which_Trav_Setup.vi"("Extra Command String"=w475) -> ("Traverse Setups"=w472:string[])
              n193 = Build Array (concatenate)(w474, w472) -> (w473:string[])
            }
            frame True {
            }
          }
        }
        n194 = call "Analyse_string_array.vi"("String array"=w428) -> ("Unique strings"=w423:string[])  [unwired: 2 out]
        n195 = for {
          tunnel: w423 -> [w440] mode=indexing
          tunnel: w427 -> [w439]
          shift-right: [w438] -> w424
          shift-left: w426 -> [w437]
          shift-right: [w435] -> w425
          shift-left: w426 -> [w436]
          n196 = stacked-sequence {
            tunnel: w440 -> [w445 w450]
            tunnel: w439 -> [w442 _]
            tunnel: [_ w449] -> w438
            tunnel: w437 -> [_ w448]
            tunnel: w436 -> [_ w447]
            tunnel: [_ w446] -> w435
            frame #0 {
              n197 = call "3D_Traverse_move.vi"("Mode"=Trav_mode."Read traverse position", "Work in Tunnel Coordinates"=w442, "Home"=Home."Don't Home", "Simulate/Run"=User_Specific_mode."Run VI", "Traverse name"=w445) -> ()  [unwired: 5 in, 6 out]
            }
            frame #1 {
              n198 = global read "DriveConfigGlobal.vi" "Configurations"() -> (w451:T22[])
              n199 = for {
                tunnel: w451 -> [w461] mode=indexing
                tunnel: w450 -> [w458]
                shift-right: [w456] -> w449
                shift-left: w448 -> [w457]
                shift-right: [w452] -> w446
                shift-left: w447 -> [w453]
                i -> [w460]
                n200 = Unbundle By Name(w461) -> ("Channel Properties.Metadata Ch Name"=w455:string)
                n201 = Format Into String(format string="%d", initial string=w458, w460) -> (resulting string=w454:string)  [unwired: 1 in, 1 out]
                n202 = Build Array (concatenate)(w457, w455) -> (w456:string[])
                n203 = Build Array (concatenate)(w453, w454) -> (w452:string[])
              }
            }
          }
        }
        n204 = global write "Trav_pos_global.vi" "ADAM Positions Ch names"(w424) -> ()
        n205 = global write "Route_mapping_global.vi" "Display Mode"("Display Mode") -> ()
        n206 = global write "Trav_pos_global.vi" "Route checking Chs"(w425) -> ()
        n207 = global write "Trav_pos_global.vi" "Traverses to Move"(w423) -> ()
      }
      frame "Initialise Measurement Prog" {
        n208 = for {
          tunnel: w484 -> [w488] mode=indexing
          tunnel: [w487] -> w478 mode=indexing
          n209 = Unbundle By Name(w488) -> ("Meas Setup File"=w487:string)
        }
        n210 = call "Analyse_string_array.vi"("String array"=w478) -> ("Unique strings"=w477:string[])  [unwired: 1 in, 1 out]
        n211 = call "Perform_Meas_Setup.vi"("Simulate/Run"=User_Specific_mode."Check VI only", "String array"=w477) -> ("Continue?"=w479:bool)  [unwired: 1 out]
        n212 = Select(t=w482, s=w479, f=Multi_Run_Case."End" ("Multi Run Case")) -> (s? t:f=w481:T3)
      }
      frame "Input Current Position" {
        n213 = call "Save_ADAM_Table_Locally.vi"() -> ()  [unwired: 12 in]
      }
      frame "Experimental setup control" {
        n214 = global read "Trav_pos_global.vi" "Source Control?"() -> (w496:bool)
        n215 = Equal?(x=w499, y=User_Specific_mode."Run VI" ("Simulate/Run")) -> (x = y?=w498:bool)
        n216 = Or(x=w496, y=w498) -> (x .or. y?=w497:bool)
        n217 = case shown="True" w497 {
          tunnel: w496 -> [_ w503]
          frame False {
          }
          frame True {
            n218 = call "Exp_Setup_Control_remote.vi"("Dispersion?"=w503) -> ()  [unwired: 3 out]
          }
        }
        n219 = global write "Trav_pos_global.vi" "FFID Background"(T6 {"Start X"=nan, "Start Y"=nan, "Start Z"=nan, "End X"=nan, "End Y"=nan, "End Z"=nan, "No. of pts."=0, "Spacing"=enum."Linear", "Filename"=path "", "Tunnel Speed"=nan, "Averaging time (min)"=nan, "Extra Commands"="", "Specific Arguments"="", "Emission Rate (l/min)"=nan, "Trace Gas Concentration (%)"=nan, "Density Ratio"="", "Comments"="", "Row No"=0, "Row Type Selector"=enum."Blank Row", "Completion time"="", "Row Duration (mins)"=nan, "No. of Valid pts."=0, "Meas Setup File"=""} ("FFID Background")) -> ()
      }
      frame "Check source flowrates" {
        n220 = case shown="\"Check VI only\", Default" w504 {
          tunnel: w505 -> [_ w514]
          frame "Check VI only", Default {
            n221 = Get Date/Time In Seconds() -> (seconds since 1Jan1904=w513:timestamp)
            n222 = global write "Trav_pos_global.vi" "Simulation Time"(w513) -> ()
          }
          frame "Run VI" {
            n223 = for {
              tunnel: w514 -> [w515] mode=indexing
              n224 = call "Set_Source.vi"("Source Status"=Client_Source_Status."Using", "Traverse line"=w515, "Simulate/Run"=User_Specific_mode."Check VI only") -> ()  [unwired: 1 in, 6 out]
            }
          }
        }
        n225 = Equal?(x=w504, y=User_Specific_mode."Run VI" ("Simulate/Run")) -> (x = y?=w508:bool)
        n226 = Increment(x=w510) -> (x+1=w506:T3)
        n227 = Select(t=w510, s=w508, f=w506) -> (s? t:f=w507:T3)
      }
      frame "Setup for running mode" {
        n228 = stacked-sequence {
          seq-local: [_ _ _ _ _ w574 _] -> [_ _ _ _ _ _ w592]
          tunnel: w521 -> [_ w549 _ _ w573 _ _]
          tunnel: w520 -> [_ _ _ w568 _ _ _]
          tunnel: [_ _ _ _ w571 _ _] -> w519
          tunnel: [_ _ _ _ _ w574 _] -> w518
          frame #0 {
            n229 = global read "Preference_global.vi" "Rig Setup"() -> (w525:string)
            n230 = Equal?(x=w525, y="EnFlo_Tunnel") -> (x = y?=w524:bool)
            n231 = case shown="True" w524 {
              frame False {
              }
              frame True {
                w535 = "EnFlo_Tunnel:Inlet_Fans:Enable"
                n232 = Build Array("EnFlo_Tunnel:Motor:Enable", w535) -> (w537:string[])
                n233 = call "Get_Current_Scan_client.vi"("ADAM Ch Names"=w537) -> ("Numerical Values"=w536:dbl[])  [unwired: 3 out]
                n234 = Index Array(array=w536) -> (element #1=w531:dbl, element #2=w532:dbl)  [unwired: 2 in]
                n235 = Less?(x=w532, y=0.5) -> (x < y?=w528:bool)
                n236 = Greater?(x=w531, y=0.5) -> (0:w529:bool)
                n237 = And(x=w529, y=w528) -> (x .and. y?=w527:bool)
                n238 = case shown="True" w527 {
                  tunnel: w535 -> [_ w538]
                  frame False {
                  }
                  frame True {
                    n239 = Format Into String(format string="The \"%s\" are not running. Do you want to put them on?", w538) -> (resulting string=w542:string)  [unwired: 2 in, 1 out]
                    n240 = Two Button Dialog(message=w542, 1:"No" ("F button name (\"Cancel\")"), 2:"Yes" ("T button name (\"OK\")")) -> (T button?=w539:bool)
                    n241 = case shown="True" w539 {
                      tunnel: w538 -> [_ w545]
                      frame False {
                      }
                      frame True {
                        n242 = Build Array(w545) -> (w546:string[])
                        n243 = call "ASYNC_Adam_client.vi"("Values"=dbl[] [1.0], "Channel Names"=w546) -> ()  [unwired: 1 in, 2 out]
                      }
                    }
                  }
                }
              }
            }
          }
          frame #1 {
            n244 = for {
              tunnel: w549 -> [w553] mode=indexing
              tunnel: [w550] -> w548 mode=indexing
              n245 = Unbundle By Name(w553) -> ("Row Type Selector"=w552:T8)
              n246 = Equal?(x=Multi_run_mode."Synchronize With:" ("Row Type Selector"), y=w552) -> (x = y?=w550:bool)
            }
            n247 = call "Setup_Environment.vi"() -> ()  [unwired: 1 in, 1 out]
            n248 = Or Array Elements(Boolean array=w548) -> (logical OR=w547:bool)
            n249 = case shown="True" w547 {
              frame False {
              }
              frame True {
                n250 = call "Declare_Sync_Client.vi"() -> ()  [unwired: 6 out]
              }
            }
          }
          frame #2 {
            n251 = Open VI Reference(vi path="Display_Trav_Views.vi" ("VI path")) -> (vi reference=w559:refnum<vi>, error out=w558:errorcluster)  [unwired: 1 in, 4 out]
            n252 = global write "Meas_global.vi" "Post Process"(Post_Process."Take New Data" ("Post Process")) -> ()
            n253 = property class="VI"(reference=w559, error in=w558, "Front Panel Window:Open"=FALSE) -> (reference out=w556:refnum<vi>, error out=w555:errorcluster)
            n254 = Close Reference(reference=w556, error in (no error)=w555) -> ()  [unwired: 1 out]
          }
          frame #3 {
            w563 = TRUE  # Start of Multi Run Prog
            w569 = TRUE
            n255 = Get Date/Time In Seconds() -> (seconds since 1Jan1904=w562:timestamp)
            n256 = To Double Precision Float(number=w562) -> (double precision float=w561:dbl)
            n257 = global write "Preference_global.vi" "Unblock Email"(w569) -> ()
            n258 = global write "Preference_global.vi" "Unblock SMS"(w569) -> ()
            n259 = global write "Meas_global.vi" "Start Time of experiment"(w561) -> ()
            n260 = local read "Command filename"() -> (w567:path)
            n261 = Path To String(path=w567) -> (string=w565:string)
            n262 = Concatenate Strings("Commencing a new multi run Prog having the setup filename of :" ("Message"), w565) -> (w564:string)
            n263 = call "Log_Current_row_to_Execute.vi"("Simulate/Run"=w568, "Message"=w564, "Start of Multi Run Prog"=w563) -> ()  [unwired: 2 in, 5 out]
          }
          frame #4 {
            n264 = call "Calc_Remaining_Time.vi"("Currently on Row"=-1, "Table In"=w573) -> ("Estimated Completion time"=w570:string, "Table Out"=w571:T6[])
            n265 = local write "Estimated Completion time"(w570) -> ()
            n266 = global write "Trav_pos_global.vi" "Estimated Completion time"(w570) -> ()
          }
          frame #5 {
            n267 = global read "Trav_pos_global.vi" "Source Control?"() -> (w575:bool)
            n268 = case shown="True" w575 {
              tunnel: [TRUE ("T button?") w580] -> w574
              frame False {
              }
              frame True {
                w581 = "EnFlo_Tunnel:Gas Solenoid:Status"
                n269 = Build Array(w581) -> (w584:string[])
                n270 = call "Get_Current_Scan_client.vi"("ADAM Ch Names"=w584) -> ("Numerical Values"=w583:dbl[])  [unwired: 3 out]
                n271 = Index Array(array=w583, index=0) -> (element=w579:dbl)
                n272 = Greater?(x=w579, y=0.5) -> (0:w577:bool)
                n273 = case shown="False" w577 {
                  tunnel: w581 -> [w590 _]
                  tunnel: [w585 TRUE ("T button?")] -> w580
                  frame False {
                    n274 = Format Into String(format string="The \"%s\" ADAM channel is showing that the blue gas button is not on.", w590) -> (resulting string=w588:string)  [unwired: 2 in, 1 out]
                    n275 = Two Button Dialog(message=w588, 1:"Stop" ("F button name (\"Cancel\")"), 2:"Continue" ("T button name (\"OK\")")) -> (T button?=w585:bool)
                  }
                  frame True {
                  }
                }
              }
            }
          }
          frame #6 {
            n276 = case shown="True" w592 {
              frame False {
              }
              frame True {
                n277 = call "Program_Active_Client.vi"("Mode"=enum16{"Program Active", "Traverse Level State"}."Traverse Level State", "Traverse level State"=Traverse_Level_State."Running") -> ()  [unwired: 1 in, 3 out]
              }
            }
          }
        }
      }
      frame "Skip Blank Rows" {
        n278 = stacked-sequence {
          tunnel: w599 -> [w602 w621]
          tunnel: w596 -> [w600 w617]
          frame #0 {
            n279 = Decrement(x=w602) -> (x-1=w601:i32)
            n280 = while {
              tunnel: w600 -> [w612]
              tunnel: w601 -> [w606]
              stop <- w603 continue-if-true
              n281 = local read "Currently on Row"() -> (w608:i32)
              n282 = Increment(x=w608) -> (x+1=w607:i32)
              n283 = Less?(x=w607, y=w606) -> (x < y?=w605:bool)
              n284 = Index Array(array=w612, index=w607) -> (element=w611:T6)
              n285 = Unbundle By Name(w611) -> ("Row Type Selector"=w610:T8)
              n286 = Equal?(x=Multi_run_mode."Blank Row" ("Row Type Selector"), y=w610) -> (x = y?=w604:bool)
              n287 = case shown="True" w604 {
                tunnel: w607 -> [_ w613]
                frame False {
                }
                frame True {
                  n288 = local write "Currently on Row"(w613) -> ()
                }
              }
              n289 = And(x=w604, y=w605) -> (x .and. y?=w603:bool)
            }
          }
          frame #1 {
            n290 = local read "Currently on Row"() -> (w619:i32)
            n291 = Increment(x=w619) -> (x+1=w618:i32)
            n292 = Index Array(array=w617, index=w618) -> (element=w620:T6)
            n293 = Unbundle By Name(w620) -> ("Row Type Selector"=w616:T8)
            n294 = Equal?(x=Multi_run_mode."Turn Off Row Repeating" ("Row Type Selector"), y=w616) -> (x = y?=w614:bool)
            n295 = while {
              shift-right: [w630] -> _
              shift-left: _ -> [w629]
              tunnel: w621 -> [w626]
              tunnel: w619 -> [w630]
              tunnel: w614 -> [w623]
              stop <- TRUE stop-if-true
              n296 = Decrement(x=w626) -> (x-1=w631:i32)
              n297 = Equal?(x=w630, y=w631) -> (x = y?=w624:bool)
              n298 = Not Equal?(x=w630, y=w629) -> (x != y?=w628:bool)
              n299 = Or(x=w623, y=w624) -> (x .or. y?=w622:bool)
              n300 = And(x=w628, y=w622) -> (x .and. y?=w627:bool)
              n301 = case shown="True" w627 {
                tunnel: w626 -> [_ w632]
                frame False {
                }
                frame True {
                  n302 = Initialize Array(timestamp(0 s since 1904-01-01) ("seconds since 1Jan1904"), w632) -> (w634:timestamp[])
                  n303 = global write "Trav_pos_global.vi" "Row completion times"(w634) -> ()
                }
              }
            }
          }
        }
      }
      frame "Which row to execute next" {
        # "Rep?"
        # "Repeat\nRow"
        n304 = local read "Currently on Row"() -> (w635:i32)
        n305 = stacked-sequence {
          seq-local: [_ w674 _] -> [_ _ w710]
          seq-local: [_ w673 _] -> [_ _ w711]
          seq-local: [w644 _ _] -> [_ w672 _]
          seq-local: [_ w669 _] -> [_ _ w704]
          tunnel: [w649 _ _] -> w641
          tunnel: w640 -> [w649 w676 w718]
          tunnel: w639 -> [_ _ w716]
          tunnel: w638 -> [_ w671 w717]
          tunnel: [_ _ w713] -> w637
          tunnel: w636 -> [_ _ w712]
          tunnel: w635 -> [w646 w668 w703]
          frame #0 {
            n306 = Array Size(array=w649) -> (size(s)=w648:i32)
            n307 = Decrement(x=w648) -> (x-1=w647:i32)
            n308 = Increment(x=w646) -> (x+1=w645:i32)
            n309 = while {
              tunnel: w645 -> [w653]
              tunnel: w649 -> [w665] mode=indexing
              tunnel: Multi_run_mode."Turn Off Row Repeating" ("Row Type Selector") -> [w664]
              tunnel: w647 -> [w660]
              tunnel: [w655] -> w644
              i -> [w657]
              stop <- w663 continue-if-true
              n310 = Less?(x=w657, y=w653) -> (x < y?=w658:bool)
              n311 = Unbundle By Name(w665) -> ("Row Type Selector"=w662:T8)
              n312 = Less?(x=w657, y=w660) -> (x < y?=w659:bool)
              n313 = Equal?(x=w657, y=w653) -> (x = y?=w654:bool)
              n314 = Equal?(x=w664, y=w662) -> (x = y?=w656:bool)
              n315 = case shown="True" w656 {
                tunnel: [TRUE w667] -> w655
                tunnel: w654 -> [_ w667]
                frame False {
                }
                frame True {
                }
              }
              n316 = Not(x=w656) -> (.not. x?=w661:bool)
              n317 = Compound Arithmetic op=AND(w661, w658, w659) -> (w663:bool)
            }
            n318 = global write "Trav_pos_global.vi" "Currently on point"(0 ("Currently on point")) -> ()
            n319 = global write "Trav_pos_global.vi" "Paused During Row?"(FALSE ("Paused During Row?")) -> ()
            n320 = global write "Trav_pos_global.vi" "Repeat Rows?"(w644) -> ()
          }
          frame #1 {
            n321 = global read "Trav_pos_global.vi" "Row completion times"() -> (w675:timestamp[])
            n322 = global read "Extra_Commands_Global.vi" "Minutes Before Repeating Row"() -> (w670:string)
            n323 = case shown="\"Run VI\"" w671 {
              tunnel: [w677 w678] -> w669
              frame "Check VI only" {
                n324 = global read "Trav_pos_global.vi" "Simulation Time"() -> (w677:timestamp)
              }
              frame "Run VI" {
                n325 = Get Date/Time In Seconds() -> (seconds since 1Jan1904=w678:timestamp)
                n326 = global write "Trav_pos_global.vi" "Simulation Time"(w678) -> ()
              }
            }
            n327 = while {
              tunnel: w676 -> [w688] mode=indexing
              tunnel: w675 -> [w691]
              tunnel: w669 -> [w690]
              tunnel: [w681] -> w674
              tunnel: [w680] -> w673
              tunnel: w672 -> [w684]
              tunnel: w668 -> [w682]
              tunnel: w670 -> [w679]
              i -> [w680]
              stop <- w687 continue-if-true
              n328 = Unbundle By Name(w688) -> ("Extra Commands"=w692:string)
              n329 = call "Extra_Commands.vi"("String to Search"=w692, "Command"=w679) -> ("Numeric Value"=w689:dbl, "Command Found"=w685:bool)  [unwired: 1 in, 3 out]
              n330 = And(x=w684, y=w685) -> (x .and. y?=w683:bool)
              n331 = case shown="True" w683 {
                tunnel: w691 -> [_ w698]
                tunnel: w690 -> [_ w699]
                tunnel: w680 -> [_ w697]
                tunnel: w689 -> [_ w695]
                tunnel: [FALSE w694] -> w681
                frame False {
                }
                frame True {
                  n332 = Index Array(array=w698, index=w697) -> (element=w700:timestamp)
                  n333 = Subtract(x=w699, y=w700) -> (x-y=w701:dbl)
                  n334 = Divide(x=w701, y=60.0) -> (x/y=w696:dbl)
                  n335 = Greater?(x=w696, y=w695) -> (0:w694:bool)
                }
              }
              n336 = Less?(x=w680, y=w682) -> (x < y?=w686:bool)
              n337 = Compound Arithmetic op=AND(invert w681, w686) -> (w687:bool)
            }
          }
          frame #2 {
            n338 = Not Equal?(x=w703, y=w711) -> (x != y?=w709:bool)
            n339 = And(x=w710, y=w709) -> (x .and. y?=w708:bool)
            n340 = case shown="False" w708 {
              tunnel: w711 -> [_ w744]
              tunnel: w703 -> [w740 w746]
              tunnel: [w739 w745] -> w714
              tunnel: [w739 w744] -> w705
              tunnel: w716 -> [w742 _]
              tunnel: [w738 TRUE] -> w715
              frame False {
                n341 = Increment(x=w740) -> (x+1=w741:i32)
                n342 = Greater?(x=w742, y=w741) -> (0:w738:bool)
                n343 = Select(t=w741, s=w738, f=w740) -> (s? t:f=w739:i32)
              }
              frame True {
                n344 = Greater?(x=w746, y=w744) -> (0:w747:bool)
                n345 = Select(t=w746, s=w747, f=w744) -> (s? t:f=w745:i32)
              }
            }
            n346 = global read "Trav_pos_global.vi" "Row completion times"() -> (w707:timestamp[])
            n347 = case shown="True" w715 {
              tunnel: w705 -> [_ w726]
              tunnel: w718 -> [_ w732]
              tunnel: w717 -> [w720 w724]
              tunnel: w714 -> [_ w730]
              tunnel: [w719 w729] -> w713
              tunnel: w712 -> [_ w729]
              frame False {
                n348 = case shown="\"Run VI\"" w720 {
                  tunnel: [Multi_Run_Case."Show jumped positions" ("Multi Run Case") Multi_Run_Case."Shut down source etc" ("Multi Run Case")] -> w719
                  frame "Check VI only" {
                  }
                  frame "Run VI" {
                  }
                }
              }
              frame True {
                n349 = Index Array(array=w732, index=w726) -> (element=w728:T6)
                n350 = Bundle By Name(cluster=w728, "Row No"=w726) -> (w727:T6)
                n351 = global write "Trav_pos_global.vi" "Meas Setup Number"(0 ("Meas Setup Number")) -> ()
                n352 = Build Array(w730) -> (w731:i32[])
                n353 = case shown="\"Run VI\"" w724 {
                  tunnel: w724 -> [_ w736]
                  tunnel: w727 -> [w733 w735]
                  tunnel: [w733 w734] -> w723
                  frame "Check VI only" {
                  }
                  frame "Run VI" {
                    n354 = call "Log_Current_row_to_Execute.vi"("Simulate/Run"=w736, "Start of Multi Run Prog"=FALSE, "Traverse line in"=w735) -> ("Traverse line Out"=w734:T6)  [unwired: 2 in, 4 out]
                  }
                }
                n355 = property on="Table" class="Arr (strict)"("Index Values"=w731) -> ()  [unwired: 2 in, 2 out]
                n356 = global write "Trav_pos_global.vi" "Current Row"(w723) -> ()
                "Currently on Row" <- w730
              }
            }
            n357 = Replace Array Subset(array=w707, new element=w704, index=w705) -> (w706:timestamp[])
            n358 = global write "Trav_pos_global.vi" "Row completion times"(w706) -> ()
          }
        }
      }
      frame "Evaluate IF Statement" {
        n359 = global read "Trav_pos_global.vi" "Current Row"() -> (w752:T6)
        n360 = Unbundle By Name(w752) -> ("Extra Commands"=w755:string)
        n361 = global read "Extra_Commands_Global.vi" "If Command"() -> (w758:string)
        n362 = call "Extra_Commands.vi"("String to Search"=w755, "Command"=w758) -> ("String Value"=w757:string, "Command Found"=w749:bool)  [unwired: 1 in, 3 out]
        n363 = Equal?(x=w753, y=User_Specific_mode."Run VI" ("Simulate/Run")) -> (x = y?=w748:bool)
        n364 = And(x=w749, y=w748) -> (x .and. y?=w750:bool)
        n365 = case shown="True" w750 {
          tunnel: w757 -> [_ w768]
          tunnel: [w764 w767] -> w751
          frame False {
            w764 = TRUE  # Execute Row?
          }
          frame True {
            n366 = call "Get_array_values_fr_String.vi"("String Value"=w768) -> ("Numeric Array"=w766:dbl[], "String array"=w765:string[])
            n367 = Index Array(array=w765, index=0 ("Index")) -> (element=w769:string)
            n368 = case shown="\"Global Value Between\"" w769 {
              tunnel: w768 -> [w774 _ _ _]
              tunnel: [w773 w775 w785 TRUE ("Execute Row?")] -> w767
              tunnel: w766 -> [_ w781 w799 _]
              tunnel: w765 -> [_ _ w793 _]
              frame "Time Between" {
                n369 = Get Date/Time In Seconds() -> (seconds since 1Jan1904=w771:timestamp)
                n370 = To Double Precision Float(number=w771) -> (double precision float=w772:dbl)
                n371 = call "If_Time_arguments.vi"("seconds since 1Jan1904"=w772, "String Value"=w774) -> ("Execute Row?"=w773:bool)  [unwired: 2 out]
              }
              frame "Global Value Between" {
                n372 = global read "Extra_Commands_Global.vi" "If command global value"() -> (w776:dbl)
                n373 = Index Array(array=w781, index=1 ("Index")) -> (element=w779:dbl)
                n374 = Index Array(array=w781, index=2 ("Index")) -> (element=w780:dbl)
                n375 = Max & Min(x=w779, y=w780) -> (max(x,y)=w778:dbl, min(x,y)=w777:dbl)
                n376 = In Range and Coerce(upper limit=w778, x=w776, lower limit=w777) -> (In Range?=w775:bool)  [unwired: 1 out]
              }
              frame "ADAM Channel Between" {
                n377 = Index Array(array=w793, index=1 ("Index")) -> (element=w792:string)
                n378 = Build Array(w792) -> (w791:string[])
                n379 = Index Array(array=w799, index=2 ("Index")) -> (element=w797:dbl)
                n380 = Index Array(array=w799, index=3 ("Index")) -> (element=w798:dbl)
                n381 = Max & Min(x=w797, y=w798) -> (max(x,y)=w796:dbl, min(x,y)=w795:dbl)
                n382 = call "Get_Current_Scan_client.vi"("ADAM Ch Names"=w791) -> ("Numerical Values"=w789:dbl[])  [unwired: 3 out]
                n383 = Index Array(array=w789, index=0 ("Index")) -> (element=w788:dbl)
                n384 = In Range and Coerce(upper limit=w796, x=w788, lower limit=w795) -> (In Range?=w786:bool)  [unwired: 1 out]
                n385 = Not A Number/Path/Refnum?(number/path/refnum=w788) -> (NaN/Path/Refnum?=w787:bool)
                n386 = Select(t=TRUE, s=w787, f=w786) -> (s? t:f=w785:bool)
              }
              frame "No Match", Default {
              }
            }
          }
        }
        n387 = Select(t=w761, s=w751, f=Multi_Run_Case."Calculate Row TIme" ("Multi Run Case")) -> (s? t:f=w760:T3)
      }
      frame "Perform Measurement Setup" {
        n388 = global read "Trav_pos_global.vi" "Current Row"() -> (w805:T6)
        n389 = case shown="\"Run VI\"" w804 {
          tunnel: w805 -> [_ w810]
          tunnel: w804 -> [_ w809]
          frame "Check VI only" {
          }
          frame "Run VI" {
            n390 = stacked-sequence {
              tunnel: w810 -> [w813 _]
              tunnel: w809 -> [w811 _]
              frame #0 {
                n391 = Unbundle By Name(w813) -> ("Extra Commands"=w812:string)
                n392 = call "Pause_for_server_ch_val.vi"("Extra command string"=w812, "Simulate/Run"=w811) -> ()  [unwired: 2 out]
              }
              frame #1 {
                n393 = Get Date/Time In Seconds() -> (seconds since 1Jan1904=w814:timestamp)
                n394 = To Double Precision Float(number=w814) -> (double precision float=w815:dbl)
                n395 = global write "Trav_pos_global.vi" "Start of Row time (Sec)"(w815) -> ()
              }
            }
          }
        }
      }
      frame "Set Measurement Conditions" {
        w821 = TRUE  # Row Completed
        w820 = FALSE  # Row Completed
        n396 = global read "Trav_pos_global.vi" "Current Row"() -> (w818:T6)
        n397 = Unbundle By Name(w818) -> ("Row Type Selector"=w823:T8)
        n398 = case shown="\"Send Message\"" w823 {
          tunnel: [TRUE FALSE TRUE TRUE TRUE TRUE FALSE TRUE FALSE w872 FALSE FALSE FALSE] -> w828
          tunnel: w818 -> [w836 w839 w842 w845 w848 w851 w854 w857 w866 w871 w896 w899 w902]
          tunnel: [w836 w839 w842 w845 w848 w851 w854 w857 w865 w870 w896 w899 w902] -> w824
          tunnel: [w835 w838 w841 w844 w847 w850 w853 w856 w861 w868 w895 w898 w901] -> w822
          tunnel: w821 -> [w835 _ w841 w844 w847 _ _ _ _ w868 w895 w898 w901]
          tunnel: w820 -> [_ w838 _ _ _ w850 w853 w856 w861 _ _ _ _]
          tunnel: w817 -> [_ _ _ _ _ _ _ _ _ w869 _ _ _]
          frame "Move Traverse Only" {
          }
          frame "Check Beam Power" {
          }
          frame "Set Tunnel Speed Only" {
          }
          frame "Set Source Only" {
          }
          frame "Set Measurement Conditions" {
          }
          frame "Single Measurement" {
          }
          frame "Vertical Profile", Default {
          }
          frame "Scanning Valve Measurement" {
          }
          frame "Run VI Named:" {
            n399 = global read "Extra_Commands_Global.vi" "Skip Source Demand"() -> (w864:string)
            n400 = global read "Extra_Commands_Global.vi" "Establish Exp Conditions (s)"() -> (w860:string)
            n401 = Unbundle By Name(w866) -> ("Extra Commands"=w863:string)
            n402 = Concatenate Strings(w860, " = 0" ("Substring"), w864, w863) -> (w862:string)
            n403 = Bundle By Name(cluster=w866, "Extra Commands"=w862) -> (w865:T6)
          }
          frame "Send Message" {
            n404 = stacked-sequence {
              seq-local: [w873 _ _ _] -> [_ w881 _ _]
              tunnel: [_ _ _ FALSE] -> w872
              tunnel: w871 -> [_ w883 w889 w892]
              tunnel: [_ _ _ w892] -> w870
              tunnel: w869 -> [w874 _ _ _]
              frame #0 {
                n405 = Equal?(x=User_Specific_mode."Run VI" ("Simulate/Run"), y=w874) -> (x = y?=w873:bool)
              }
              frame #1 {
                n406 = Unbundle By Name(w883) -> ("Specific Arguments"=w877:string, "Comments"=w878:string, "Filename"=w880:path)
                n407 = Concatenate Strings(w877, w878) -> (w876:string)
                n408 = Build Array(w880) -> (w879:path[])
                n409 = case shown="True" w881 {
                  tunnel: "Message" ("Error Type") -> [_ w886]
                  tunnel: w876 -> [_ w885]
                  tunnel: w879 -> [_ w884]
                  frame False {
                  }
                  frame True {
                    n410 = call "Email_Text_Files.vi"("Filenames"=w884, "message"=w885, "subject ([No Subject])"=w886) -> ()
                  }
                }
              }
              frame #2 {
                n411 = global read "Extra_Commands_Global.vi" "Establish Exp Conditions (s)"() -> (w891:string)
                n412 = Unbundle By Name(w889) -> ("Extra Commands"=w890:string)
                n413 = call "Extra_Commands.vi"("String to Search"=w890, "Command"=w891) -> ("Numeric Value"=w887:dbl)  [unwired: 1 in, 4 out]
                n414 = call "Wait_Seconds_with_display.vi"("Message"="In Send Message Row", "Seconds to wait"=w887) -> ()  [unwired: 2 out]
              }
              frame #3 {
              }
            }
          }
          frame "Fall Back to this Row" {
          }
          frame "Turn Off Row Repeating" {
          }
          frame "Blank Row" {
          }
        }
        n415 = case shown="True" w828 {
          tunnel: w824 -> [_ w904]
          tunnel: w817 -> [_ w908]
          tunnel: [Multi_Run_Status."Continue" ("Status") w905] -> w816
          frame False {
          }
          frame True {
            w907 = 1  # Currently on Point
            n416 = call "Program_Active.vi"() -> ()  [unwired: 1 in]
            n417 = call "Set_Measurement_Conditions.vi"("Simulate/Run"=w908, "Currently on Point"=w907, "Traverse line"=w904) -> ("Status Cluster"=w906:T25)  [unwired: 2 out]
            n418 = Unbundle By Name(w906) -> ("Status"=w905:T2)
          }
        }
        n419 = case shown="\"Continue\"" w816 {
          tunnel: [w832 Multi_Run_Case."Calculate Row TIme" ("Multi Run Case")] -> w827
          tunnel: w826 -> [w833 _]
          tunnel: w822 -> [w830 _]
          frame "Continue" {
            n420 = Select(t=Multi_Run_Case."Calculate Row TIme" ("Multi Run Case"), s=w830, f=w833) -> (s? t:f=w832:T3)
          }
          frame "Jump to Next Point", Default {
          }
        }
        n421 = local write "Status"(w816) -> ()
      }
      frame "Execute Row" {
        n422 = global read "Trav_pos_global.vi" "Current Row"() -> (w910:T6)
        n423 = stacked-sequence {
          tunnel: w911 -> [w915 w926 w928]
          tunnel: w910 -> [w916 w923 w927]
          frame #0 {
            n424 = case shown="\"Check VI only\"" w915 {
              tunnel: w916 -> [w919 _]
              tunnel: w915 -> [w918 _]
              frame "Check VI only" {
                n425 = Unbundle By Name(w919) -> ("Extra Commands"=w920:string, "Row No"=w922:i32, "Meas Setup File"=w917:string)
                n426 = call "Skip_If Sd_Error_Below.vi"("String to Search"=w920, "Simulate/Run"=w918, "Measurement setup Applied?"=TRUE, "Row Number"=w922, "Measurement Setup File"=w917) -> ()  [unwired: 5 out]
              }
              frame "Run VI" {
              }
            }
          }
          frame #1 {
            n427 = call "Execute_Row.vi"("Simulate/Run"=w926, "Traverse line"=w923) -> ("Status"=w925:T2, "Traverse line out"=w924:T6)  [unwired: 2 out]
            n428 = local write "Status"(w925) -> ()
            n429 = global write "Trav_pos_global.vi" "Current Row"(w924) -> ()
          }
          frame #2 {
            w931 = FALSE  # Empty list
            n430 = call "Remember_RD_Folders.vi"("Empty list"=w931) -> ("List of Folders"=w930:path[])  [unwired: 1 in]
            n431 = for {
              tunnel: w927 -> [w936]
              tunnel: w930 -> [w935] mode=indexing
              tunnel: "Muti_Run_Log.xls" ("name or relative path") -> [w933]
              tunnel: w928 -> [w932]
              n432 = Build Path(base path=w935, name or relative path=w933) -> (appended path=w934:path)
              n433 = call "Log_Current_row_to_Execute.vi"("Simulate/Run"=w932, "Start of Multi Run Prog"=FALSE, "Traverse line in"=w936, "Multi Run Log File"=w934) -> ()  [unwired: 1 in, 5 out]
            }
          }
        }
      }
      frame "Calculate Row TIme" {
        n434 = global read "Trav_pos_global.vi" "Paused During Row?"() -> (w941:bool)
        n435 = local read "Status"() -> (w944:T2)
        n436 = global read "Trav_pos_global.vi" "Current Row"() -> (w940:T6)
        n437 = Equal?(x=w944, y=Multi_Run_Status."Continue" ("Status")) -> (x = y?=w943:bool)
        n438 = Equal?(x=w946, y=User_Specific_mode."Run VI" ("Simulate/Run")) -> (x = y?=w942:bool)
        n439 = Compound Arithmetic op=AND(w943, w942, invert w941) -> (w939:bool)
        n440 = case shown="False" w939 {
          tunnel: w940 -> [w959 w970]
          frame False {
            n441 = global read "Trav_pos_global.vi" "Simulation Time"() -> (w960:timestamp)
            n442 = To Double Precision Float(number=w960) -> (double precision float=w954:dbl)
            n443 = call "Calculate_Row_Time.vi"("Row Start Time (Sec Since 1904)"=w954, "Multi Run Row"=w959) -> ("Scalable Time (Sec)"=w957:dbl, "Fixed Time (Sec)"=w955:dbl)
            n444 = call "Overhead_Factor.vi"("Mode"=Overhead."Read Current Overhead") -> ("Current Overhead Factor"=w958:dbl)  [unwired: 3 in]
            n445 = Multiply(x=w958, y=w957) -> (x*y=w956:dbl)
            n446 = Add(x=w955, y=w956) -> (x+y=w951:dbl)
            n447 = global write "Trav_pos_global.vi" "Start of Row time (Sec)"(w951) -> ()
            n448 = Add(x=w954, y=w951) -> (x+y=w953:dbl)
            n449 = To Time Stamp(1:w953) -> (0:w952:timestamp)
            n450 = global write "Trav_pos_global.vi" "Simulation Time"(w952) -> ()
          }
          frame True {
            n451 = global read "Trav_pos_global.vi" "Start of Row time (Sec)"() -> (w968:dbl)
            n452 = Get Date/Time In Seconds() -> (seconds since 1Jan1904=w963:timestamp)
            n453 = To Double Precision Float(number=w963) -> (double precision float=w962:dbl)
            n454 = call "Calculate_Row_Time.vi"("Row Start Time (Sec Since 1904)"=w968, "Multi Run Row"=w970) -> ("Scalable Time (Sec)"=w964:dbl, "Fixed Time (Sec)"=w966:dbl)
            n455 = Subtract(x=w962, y=w968) -> (x-y=w967:dbl)
            n456 = Subtract(x=w967, y=w966) -> (x-y=w965:dbl)
            n457 = call "Overhead_Factor.vi"("Sum of Ideal times (Sec)"=w964, "Sum of Actual times (Sec)"=w965, "Mode"=Overhead."Update total times") -> ()  [unwired: 1 in, 1 out]
          }
        }
      }
      frame "Update time estimate" {
        n458 = global read "Trav_pos_global.vi" "Current Row"() -> (w974:T6)
        n459 = Unbundle By Name(w974) -> ("Row No"=w972:i32)
        n460 = local read "Currently on Row"() -> (w973:i32)
        n461 = Equal?(x=w972, y=w973) -> (x = y?=w971:bool)
        n462 = case shown="\"Run VI\"" w977 {
          tunnel: w980 -> [w988 w1011]
          tunnel: [w987 w1007] -> w979
          tunnel: w976 -> [_ w1013]
          tunnel: [w986 w1012] -> w975
          tunnel: w973 -> [w984 w1006]
          tunnel: w974 -> [w985 w1010]
          tunnel: w971 -> [w983 w1009]
          frame "Check VI only" {
            n463 = global read "Trav_pos_global.vi" "Simulation Time"() -> (w990:timestamp)
            n464 = To Double Precision Float(number=w990) -> (double precision float=w989:dbl)
            n465 = call "Sec_to_date_filename.vi"("seconds"=w989) -> ("Day"=w992:string, "Time"=w991:string)  [unwired: 2 out]
            n466 = Concatenate Strings(w991, "  " ("Substring"), w992) -> (w986:string)
            n467 = case shown="True" w983 {
              tunnel: w984 -> [_ w1003]
              tunnel: w988 -> [w994 w1002]
              tunnel: [w994 w1000] -> w987
              tunnel: w986 -> [_ w999]
              tunnel: w985 -> [_ w998]
              frame False {
              }
              frame True {
                n468 = global read "Trav_pos_global.vi" "Start of Row time (Sec)"() -> (w997:dbl)
                n469 = Divide(x=w997, y=60.0) -> (x/y=w995:dbl)
                n470 = Bundle By Name(cluster=w998, "Completion time"=w999, "Row Duration (mins)"=w995) -> (w1001:T6)
                n471 = Replace Array Subset(array=w1002, new element=w1001, index=w1003) -> (w1000:T6[])
              }
            }
          }
          frame "Run VI" {
            n472 = case shown="True" w1009 {
              tunnel: w1006 -> [_ w1020]
              tunnel: w1011 -> [w1016 w1019]
              tunnel: w1010 -> [_ w1018]
              tunnel: [w1016 w1017] -> w1008
              frame False {
              }
              frame True {
                n473 = Replace Array Subset(array=w1019, new element=w1018, index=w1020) -> (w1017:T6[])
              }
            }
            n474 = call "Calc_Remaining_Time.vi"("Currently on Row"=w1006, "Table In"=w1008) -> ("Table Out"=w1007:T6[])  [unwired: 1 out]
            n475 = Decrement(x=w1013) -> (x-1=w1015:i32)
            n476 = Index Array(array=w1007, index=w1015) -> (element=w1014:T6)
            n477 = Unbundle By Name(w1014) -> ("Completion time"=w1012:string)
            n478 = call "Program_Active_Client.vi"("Mode"=enum16{"Program Active", "Traverse Level State"}."Traverse Level State", "Traverse level State"=Traverse_Level_State."Running") -> ()  [unwired: 1 in, 3 out]
          }
        }
        "Estimated Completion time" <- w975
        n479 = global write "Trav_pos_global.vi" "Estimated Completion time"(w975) -> ()
      }
      frame "Pause Multi Run Program" {
        n480 = while {
          tunnel: "Pause" -> [w1032]
          tunnel: [w1035] -> w1027
          tunnel: w1026 -> [w1034]
          tunnel: w1024 -> [w1033]
          shift-right: [w1032] -> _
          shift-left: _ -> [w1031]
          stop <- TRUE stop-if-true
          n481 = case shown="True" w1032 {
            tunnel: [w1036 w1041] -> w1035
            tunnel: w1034 -> [w1036 w1039]
            tunnel: w1033 -> [_ w1040]
            tunnel: w1032 -> [_ w1038]
            tunnel: w1031 -> [_ w1037]
            frame False {
            }
            frame True {
              n482 = stacked-sequence {
                tunnel: w1039 -> [_ _ _ _ w1056]
                tunnel: [_ _ _ _ w1057] -> w1041
                tunnel: w1040 -> [w1043 _ _ _ _]
                tunnel: w1038 -> [_ _ _ w1052 _]
                tunnel: w1037 -> [_ _ _ w1051 _]
                frame #0 {
                  n483 = Quotient & Remainder(x=w1043, y=15) -> (x-y*floor(x/y)=w1042:i32)  [unwired: 1 out]
                  n484 = case shown="0" w1042 {
                    frame 0 {
                      n485 = Current VI's Path() -> (path=w1045:path)
                      n486 = call "Bring_to_front.vi"("path"=w1045) -> ()
                    }
                    frame 1, Default {
                    }
                  }
                }
                frame #1 {
                  n487 = global write "Trav_pos_global.vi" "Paused During Row?"(TRUE ("Paused During Row?")) -> ()
                  "Pause message" <- "Multi Run Program Paused!!!!" ("Pause message")
                }
                frame #2 {
                  n488 = property on="Pause message" class="Str"("Visible"=TRUE) -> ()  [unwired: 2 in, 2 out]
                  n489 = Wait Until Next ms Multiple(millisecond multiple=u32 1500) -> ()  [unwired: 1 out]
                }
                frame #3 {
                  n490 = Compound Arithmetic op=AND(w1052, invert w1051) -> (w1050:bool)
                  n491 = case shown="True" w1050 {
                    frame False {
                    }
                    frame True {
                      n492 = call "Program_Active_Client.vi"("Mode"=enum16{"Program Active", "Traverse Level State"}."Program Active", "Time till next contact (Sec)"=12000.0, "Traverse level State"=Traverse_Level_State."Running") -> ()  [unwired: 3 out]
                    }
                  }
                }
                frame #4 {
                  n493 = property on="Pause message" class="Str"("Visible"=FALSE) -> ()  [unwired: 2 in, 2 out]
                  n494 = Wait Until Next ms Multiple(millisecond multiple=u32 1500) -> ()  [unwired: 1 out]
                  n495 = Decrement(x=w1056) -> (x-1=w1057:T3)
                }
              }
            }
          }
        }
        n496 = call "Overhead_Factor.vi"("Mode"=Overhead."Read Current Overhead") -> ("Current Overhead Factor"=→"Current Overhead Factor":dbl)  [unwired: 3 in]
      }
      frame "Do Another Row?" {
        w1074 = Multi_Run_Status."Terminate Run" ("Status")
        n497 = case shown="False" "Stop after Repeats" {
          tunnel: [w1095 w1096] -> w1068
          tunnel: w1064 -> [_ w1097]
          frame False {
            n498 = local read "Currently on Row"() -> (w1095:i32)
            n499 = Increment(x=w1095) -> (x+1=→"Last Row Run":i32)
          }
          frame True {
            n500 = Decrement(x=w1097) -> (x-1=w1096:i32)
            n501 = local write "Currently on Row"(w1096) -> ()
          }
        }
        n502 = global read "Preference_global.vi" "Server Comms"() -> (w1063:T26)
        n503 = case shown="\"Server Link Healthy\"" w1063 {
          tunnel: [w1083 TRUE] -> w1062
          frame "Server Link Healthy" {
            n504 = Build Array("EnFlo Lab:Emergency_Stop:Happy") -> (w1086:string[])
            n505 = call "Get_Current_Scan_client.vi"("ADAM Ch Names"=w1086) -> ("Numerical Values"=w1088:dbl[])  [unwired: 1 in, 2 out]
            n506 = Index Array(array=w1088) -> (element=w1084:dbl)  [unwired: 1 in]
            n507 = Not A Number/Path/Refnum?(number/path/refnum=w1084) -> (NaN/Path/Refnum?=w1085:bool)
            n508 = case shown="False" w1085 {
              tunnel: w1084 -> [w1091 _]
              tunnel: [w1089 TRUE] -> w1083
              frame False {
                n509 = Greater?(x=w1091, y=0.5) -> (0:w1089:bool)
              }
              frame True {
              }
            }
          }
          frame "Do Not Link To Server" {
          }
        }
        n510 = case shown="True" "stop" {
          tunnel: [w1098 w1099] -> w1075
          tunnel: w1074 -> [_ w1099]
          frame False {
            n511 = local read "Status"() -> (w1098:T2)
          }
          frame True {
            n512 = local write "Status"(w1099) -> ()
          }
        }
        n513 = Not Equal?(x=w1075, y=w1074) -> (x != y?=w1073:bool)
        n514 = Increment(x=w1068) -> (x+1=w1067:i32)
        n515 = Index Array(array=w1069, index=w1067) -> (element=w1066:T6)
        n516 = Unbundle By Name(w1066) -> ("Row Type Selector"=w1072:T8)
        n517 = Equal?(x=w1072, y=Multi_run_mode."Turn Off Row Repeating" ("Row Type Selector")) -> (x = y?=w1070:bool)
        n518 = case shown="False" w1073 {
          tunnel: [w1100 w1104] -> w1060
          tunnel: w1078 -> [w1101 _]
          tunnel: w1069 -> [_ _]
          tunnel: w1075 -> [_ w1105]
          tunnel: w1070 -> [_ _]
          frame False {
            n519 = case shown="\"Run VI\"" w1101 {
              tunnel: [Multi_Run_Case."Show jumped positions" ("Multi Run Case") Multi_Run_Case."Shut down source etc" ("Multi Run Case")] -> w1100
              frame "Check VI only" {
              }
              frame "Run VI" {
              }
            }
          }
          frame True {
            n520 = case shown="\"Jump To Fall Back\"" w1105 {
              tunnel: [Multi_Run_Case."Skip Blank Rows" ("Multi Run Case") Multi_Run_Case."Find Next Fall Back Row" ("Multi Run Case")] -> w1104
              frame "Continue", Default {
              }
              frame "Jump To Fall Back" {
              }
            }
          }
        }
        n521 = case shown="False" w1062 {
          tunnel: [Multi_Run_Case."Shut down source etc" ("Multi Run Case") w1082] -> w1061
          tunnel: w1060 -> [_ w1082]
          frame False {
            n522 = local write "Status"(Multi_Run_Status."Terminate Run" ("Status")) -> ()
          }
          frame True {
          }
        }
      }
      frame "Find Next Fall Back Row" {
        n523 = local read "Currently on Row"() -> (w1109:i32)
        n524 = Increment(x=w1109) -> (x+1=w1108:i32)
        n525 = Index Array(array=w1117, index=w1109) -> (element=w1118:T6)
        n526 = Array Size(array=w1117) -> (size(s)=w1116:i32)
        n527 = Unbundle By Name(w1118) -> ("Row Type Selector"=w1112:T8)
        n528 = Greater?(x=w1116, y=w1108) -> (0:w1115:bool)
        n529 = Equal?(x=w1112, y=Multi_run_mode."Fall Back to this Row" ("Mode")) -> (x = y?=w1110:bool)
        n530 = case shown="True" w1115 {
          tunnel: [Multi_Run_Case."Skip Blank Rows" ("Multi Run Case") w1125] -> w1114
          tunnel: w1110 -> [_ w1121]
          tunnel: w1109 -> [_ w1122]
          frame False {
          }
          frame True {
            n531 = case shown="False" w1121 {
              tunnel: w1122 -> [w1127 _]
              frame False {
                n532 = Increment(x=w1127) -> (x+1=w1126:i32)
                n533 = local write "Currently on Row"(w1126) -> ()
              }
              frame True {
              }
            }
            n534 = Select(t=Multi_Run_Case."Skip Blank Rows" ("Multi Run Case"), s=w1121, f=Multi_Run_Case."Find Next Fall Back Row" ("Multi Run Case")) -> (s? t:f=w1125:T3)
          }
        }
      }
      frame "Shut down source etc" {
        n535 = for {
          tunnel: w1145 -> [w1162] mode=indexing
          tunnel: Multi_run_mode."Synchronize With:" ("Mode") -> [w1160]
          tunnel: [w1159] -> w1147 mode=indexing
          n536 = Unbundle By Name(w1162) -> ("Row Type Selector"=w1161:T8)
          n537 = Equal?(x=w1161, y=w1160) -> (x = y?=w1159:bool)
        }
        n538 = call "Overhead_Factor.vi"("Mode"=Overhead."Re Scale totals to 3 hrs") -> ()  [unwired: 3 in, 1 out]
        n539 = local read "Status"() -> (w1135:T2)
        n540 = call "Program_Active_Client.vi"("Mode"=enum16{"Program Active", "Traverse Level State"}."Traverse Level State", "Traverse level State"=Traverse_Level_State."Complete") -> ()  [unwired: 1 in, 3 out]
        n541 = global read "Meas_global.vi" "Start Time of experiment"() -> (w1143:dbl)
        n542 = Equal?(x=w1135, y=Multi_Run_Status."Terminate Run" ("Status")) -> (x = y?=w1133:bool)
        n543 = Or Array Elements(Boolean array=w1147) -> (logical OR=w1136:bool)
        n544 = Get Date/Time In Seconds() -> (seconds since 1Jan1904=w1128:timestamp)
        n545 = Compound Arithmetic op=AND(w1136, invert w1133) -> (w1137:bool)
        n546 = To Double Precision Float(number=w1128) -> (double precision float=w1144:dbl)
        n547 = case shown="True" w1137 {
          frame False {
          }
          frame True {
            n548 = global read "Preference_global.vi" "Rig Setup"() -> (w1152:string)
            n549 = Concatenate Strings(w1152, ":Program:Sync") -> (w1154:string)
            n550 = Bundle By Name(cluster=T20 {"Channel Name"="", "New Value"=0.0} ("Update Scan Value Cluster"), "Channel Name"=w1154, "New Value"=1000.0 ("Bundle Element")) -> (w1155:T20)
            n551 = Build Array(w1155) -> (w1157:T20[])
            n552 = call "Update_Current_Value_client.vi"("Update array in"=w1157) -> ()  [unwired: 1 in]
          }
        }
        n553 = Subtract(x=w1144, y=w1143) -> (x-y=w1142:dbl)
        n554 = Greater?(x=w1142, y=300.0) -> (0:w1139:bool)
        n555 = Not(x=w1139) -> (.not. x?=→"Non Starter":bool)
        n556 = Increment(x=w1131) -> (x+1=w1130:T3)
        n557 = Increment(x=w1130) -> (x+1=w1129:T3)
        n558 = Select(t=w1131, s=w1139, f=w1129) -> (s? t:f=w1140:T3)
      }
      frame "Email results to users" {
        n559 = local read "Currently on Row"() -> (w1168:i32)
        n560 = Increment(x=w1168) -> (x+1=w1163:i32)
        n561 = Split 1D Array(array=w1165, index=w1163) -> (first subarray=w1172:T6[], second subarray=w1171:T6[])
        n562 = Array Size(array=w1171) -> (size(s)=w1173:i32)
        n563 = for {
          tunnel: w1172 -> [w1188] mode=indexing
          shift-right: [w1186] -> w1174
          shift-left: string[] [] -> [w1187]
          n564 = Unbundle By Name(w1188) -> ("Row Type Selector"=w1179:T8, "Filename"=w1185:path, "Comments"=w1184:string)
          n565 = Not Equal?(x=Multi_run_mode."Auto Calibrate" ("Row Type Selector"), y=w1179) -> (x != y?=w1181:bool)
          n566 = Empty String/Path?(string/path=w1185) -> (empty?=w1182:bool)
          n567 = Compound Arithmetic op=AND(w1181, invert w1182) -> (w1180:bool)
          n568 = case shown="True" w1180 {
            tunnel: w1187 -> [w1189 w1197]
            tunnel: [w1189 w1196] -> w1186
            tunnel: w1185 -> [_ w1195]
            tunnel: w1184 -> [_ w1193]
            frame False {
            }
            frame True {
              n569 = Path To String(path=w1195) -> (string=w1194:string)
              n570 = Match Pattern(string=w1193, regular expression=" !!Program added comments") -> (after substring=w1190:string)  [unwired: 4 out]
              n571 = Concatenate Strings(w1194, w1190) -> (w1192:string)
              n572 = Build Array (concatenate)(w1197, w1192) -> (w1196:string[])
            }
          }
        }
        n573 = Equal To 0?(x=w1173) -> (x = 0?=w1164:bool)
        n574 = case shown="False" w1164 {
          tunnel: ["Having completed only some of the requested rows." ("Message") ""] -> w1169
          frame False {
          }
          frame True {
          }
        }
        n575 = call "End_of_run_messages.vi"("Message"=w1169, "Subject"="Multi Run Ended", "Attachments"=w1174) -> ()  [unwired: 1 in]
      }
      frame "Save run efficiency" {
        w1211 = FALSE  # append to file? (new file:F)
        w1210 = FALSE  # advisory dialog? (display:T)
        n576 = call "Get_IP_Number.vi"() -> ("Computer Name"=w1199:string)  [unwired: 1 out]
        n577 = Format Into String(format string="Preferences_%s.xls" ("name or relative path"), w1199) -> (resulting string=w1198:string)  [unwired: 2 in, 1 out]
        n578 = call "Setup_Filepath.vi"("Setup File Type"=Setup_Filetype."General", "Filename in"=w1198) -> ("Filename Out"=w1201:path)  [unwired: 1 out]
        n579 = call "Overhead_Factor.vi"("Mode"=Overhead."Read Current Overhead") -> ("Current Overhead Factor"=w1205:dbl)  [unwired: 3 in]
        n580 = Number To Fractional String(number=w1205, precision (6)=i16 4) -> (F-format string=w1203:string)  [unwired: 2 out]
        n581 = call "Read_Characters_From_File.ph.vi"("file path (dialog if empty)"=w1201) -> ("character string"=w1208:string)  [unwired: 1 in, 7 out]
        n582 = call "Replace_data_in_setup_string.vi"("New data string"=w1203, "Input string"=w1208, "Variable name"="Current Overhead Factor") -> ("Appended string"=w1207:string)
        n583 = call "Write_Characters_To_File.vi"("file path (dialog if empty)"=w1201, "advisory dialog? (display:T)"=w1210, "character string"=w1207, "append to file? (new file:F)"=w1211) -> ()  [unwired: 1 in, 4 out]
      }
      frame "Remove Skipped Commands" {
        n584 = for {
          tunnel: w1217 -> [w1225] mode=indexing
          tunnel: [w1224] -> w1216 mode=indexing
          n585 = Unbundle By Name(w1225) -> ("Comments"=w1223:string)
          n586 = Match Pattern(string=w1223, regular expression=" !!Program added comments") -> (before substring=w1222:string)  [unwired: 4 out]
          n587 = Bundle By Name(cluster=w1225, "Comments"=w1222) -> (w1224:T6)
        }
      }
      frame "Show jumped positions" {
        n588 = global read "Trav_pos_global.vi" "Jumped Positions"() -> (w1228:dbl[][])
        n589 = Array Size(array=w1228) -> (size(s)=w1231:i32[])
        n590 = Index Array(array=w1231, index=0) -> (element=w1227:i32)
        n591 = Greater Than 0?(x=w1227) -> (x > 0?=w1229:bool)
        n592 = case shown="True" w1229 {
          tunnel: w1228 -> [_ w1242]
          tunnel: w1227 -> [_ w1241]
          frame False {
            w1235 = TRUE  # Front Panel Window:Is Frontmost
            n593 = Current VI's Path() -> (path=w1236:path)
            n594 = Open VI Reference(vi path=w1236) -> (vi reference=w1237:refnum<vi>, error out=w1238:errorcluster)  [unwired: 1 in, 4 out]
            n595 = property class="VI"(reference=w1237, error in=w1238, "Front Panel Window:Is Frontmost"=w1235) -> (reference out=w1239:refnum<vi>, error out=w1240:errorcluster)
            n596 = Close Reference(reference=w1239, error in (no error)=w1240) -> ()  [unwired: 1 out]
          }
          frame True {
            n597 = stacked-sequence {
              tunnel: w1242 -> [w1243 w1253]
              tunnel: w1241 -> [w1247 _]
              frame #0 {
                n598 = global read "Trav_pos_global.vi" "Default Traverse Setup"() -> (w1244:string)
                n599 = Format Into String(format string="There are %d points which cannot be reached", w1247) -> (resulting string=w1245:string)  [unwired: 2 in, 1 out]
                n600 = call "Display_Trav_Views.vi"("Current Probe Position"=w1243, "Traverse Name"=w1244, "Open Front Panel"=TRUE, "Error Comments"=w1245, "Crash?"=FALSE) -> ()  [unwired: 2 in, 4 out]
              }
              frame #1 {
                n601 = local read "Command filename"() -> (w1257:path)
                n602 = Array To Spreadsheet String(array=w1253, 3:"%.1f" ("format string")) -> (spreadsheet string=w1251:string)  [unwired: 1 out]
                n603 = Strip Path(path=w1257) -> (stripped path=w1256:path)  [unwired: 1 out]
                n604 = Build Path(base path=w1256, name or relative path="Jumped_Positions.xls") -> (appended path=w1254:path)
                n605 = call "Write_File_Simple.vi"("append to file? (new file:F)"=FALSE, "character string"=w1251, "file path"=w1254) -> ()  [unwired: 2 out]
              }
            }
          }
        }
      }
      frame "Save Setup to File" {
        w1275 = FALSE  # Start of Multi Run Prog
        n606 = Array Size(array=w1289) -> (size(s)=w1294:i32)
        n607 = local read "Last Row Run"() -> (w1264:i32)
        n608 = local read "Status"() -> (w1270:T2)
        n609 = local read "Stop after Repeats"() -> (w1273:bool)
        n610 = local read "stop"() -> (w1274:bool)
        n611 = Decrement(x=w1264) -> (x-1=w1265:i32)
        n612 = local read "Command filename"() -> (w1260:path)
        n613 = Increment(x=w1265) -> (x+1=w1277:i32)
        n614 = Equal?(x=w1270, y=Multi_Run_Status."Continue" ("Status")) -> (x = y?=w1269:bool)
        n615 = Compound Arithmetic op=OR(w1273, w1274, w1269) -> (w1272:bool)
        n616 = local read "Non Starter"() -> (w1282:bool)
        n617 = Select(t=w1277, s=w1272, f=w1265) -> (s? t:f=w1276:i32)
        n618 = Less?(x=w1268, y=T9."Run Multi Run Prog") -> (x < y?=w1266:bool)
        n619 = Equal?(x=w1294, y=w1264) -> (x = y?=w1284:bool)
        n620 = Equal To 0?(x=w1277) -> (x = 0?=w1283:bool)
        n621 = Split 1D Array(array=w1289, index=w1276) -> (second subarray=w1292:T6[])  [unwired: 1 out]
        n622 = Compound Arithmetic op=OR(w1284, w1283, w1282, w1266) -> (w1285:bool)
        n623 = call "Current_Filepath.vi"("Short_Name"="Cmd" ("Data Type"), "Filename in"=w1260, "Data Type"="Commands") -> ("Filename Out"=w1259:path)  [unwired: 1 in, 1 out]
        n624 = local read "Work in Tunnel Coordinates?"() -> (w1263:T1)
        n625 = local read "Jump Bad Positions"() -> (w1262:bool)
        n626 = case shown="False" w1285 {
          tunnel: w1259 -> [w1302 w1336]
          tunnel: [w1301 w1336] -> w1293
          tunnel: w1292 -> [w1299 _]
          tunnel: [w1298 w1337] -> w1291
          tunnel: w1289 -> [w1300 w1337]
          tunnel: w1263 -> [w1297 _]
          tunnel: w1262 -> [w1296 _]
          frame False {
            n627 = stacked-sequence {
              tunnel: w1302 -> [w1304 w1315 _]
              tunnel: [_ w1308 _] -> w1301
              tunnel: w1300 -> [w1307 _ w1320]
              tunnel: w1299 -> [_ _ w1318]
              tunnel: [_ _ w1317] -> w1298
              tunnel: w1297 -> [w1306 _ _]
              tunnel: w1296 -> [w1305 _ _]
              frame #0 {
                n628 = call "Save_Trav_setup.vi"("Work in Tunnel Coordinates?"=w1306, "Trav Table"=w1307, "Jump Bad Positions"=w1305, "Setup filename"=w1304) -> ()  [unwired: 2 out]
                n629 = global write "Trav_pos_global.vi" "Sync to server now"(TRUE) -> ()
              }
              frame #1 {
                n630 = Strip Path(path=w1315) -> (stripped path=w1316:path, name=w1314:string)
                n631 = call "Add_filename_suffix.vi"("Filename"=w1314) -> ("Original Suffix"=w1311:string, "Base name"=w1313:string)  [unwired: 1 in, 2 out]
                n632 = Concatenate Strings(w1313, "_Rem", w1311) -> (w1310:string)
                n633 = Build Path(base path=w1316, name or relative path=w1310) -> (appended path=w1309:path)
                n634 = call "Find_Unique_Filename.vi"("Path In"=w1309) -> ("Unique Path Out"=w1308:path)  [unwired: 1 in, 1 out]
              }
              frame #2 {
                n635 = Index Array(array=w1320, index=0) -> (element=w1323:T6)
                n636 = Initialize Array(w1323, 0 ("dimension size")) -> (w1322:T6[])
                n637 = global read "Extra_Commands_Global.vi" "Minutes Before Repeating Row"() -> (w1321:string)
                n638 = for {
                  shift-right: [w1326] -> w1319
                  shift-left: w1322 -> [w1328]
                  tunnel: w1321 -> [w1330]
                  tunnel: w1320 -> [w1327] mode=indexing
                  n639 = Unbundle By Name(w1327) -> ("Extra Commands"=w1329:string)
                  n640 = call "Extra_Commands.vi"("String to Search"=w1329, "Command"=w1330) -> ("Command Found"=w1331:bool)  [unwired: 1 in, 4 out]
                  n641 = case shown="False" w1331 {
                    tunnel: w1328 -> [w1332 w1335]
                    tunnel: w1327 -> [_ w1334]
                    tunnel: [w1332 w1333] -> w1326
                    frame False {
                    }
                    frame True {
                      n642 = Build Array (concatenate)(w1335, w1334) -> (w1333:T6[])
                    }
                  }
                }
                n643 = Build Array (concatenate)(w1319, w1318) -> (w1317:T6[])
              }
            }
          }
          frame True {
          }
        }
        n644 = Path To String(path=w1259) -> (string=w1281:string)
        n645 = Concatenate Strings("Multi run Prog Ended having the setup filename of :" ("Message"), w1281) -> (w1280:string)
        n646 = call "Save_Trav_setup.vi"("Work in Tunnel Coordinates?"=w1263, "Trav Table"=w1291, "Jump Bad Positions"=w1262, "Setup filename"=w1293) -> ("Trav Table Out"=w1290:T6[])  [unwired: 1 out]
        n647 = call "Log_Current_row_to_Execute.vi"("Simulate/Run"=w1279, "Message"=w1280, "Start of Multi Run Prog"=w1275) -> ()  [unwired: 2 in, 5 out]
        n648 = Select(t=w1290, s=w1285, f=w1289) -> (s? t:f=w1288:T6[])
      }
      frame "End" {
        w1339 = ""
        w1341 = path ""
        w1342 = 0 ("No. of pts.")
        w1344 = nan
        n649 = global write "Trav_pos_global.vi" "Top level setup filename"(w1341) -> ()
        n650 = global read "Trav_pos_global.vi" "Current Row"() -> (w1348:T6)
        n651 = Bundle By Name(cluster=w1348, "Start X"=w1344, "Start Y"=w1344, "Start Z"=w1344, "End X"=w1344, "End Y"=w1344, "End Z"=w1344, "No. of pts."=w1342, "Spacing"=Spacing."Linear", "Filename"=w1341, "Tunnel Speed"=w1344, "Averaging time (min)"=w1344, "Extra Commands"=w1339, "Specific Arguments"=w1339, "Emission Rate (l/min)"=w1344, "Trace Gas Concentration (%)"=w1344, "Density Ratio"=w1339, "Comments"=w1339, "Row No"=w1342, "Row Type Selector"=Multi_run_mode."Blank Row", "Completion time"=w1339, "Meas Setup File"=w1339, "Row Duration (mins)"=w1344, "No. of Valid pts."=w1342) -> (w1347:T6)
        n652 = Current VI's Path() -> (path=w1340:path)
        n653 = global write "Trav_pos_global.vi" "Current Row"(w1347) -> ()
        n654 = global write "Trav_pos_global.vi" "Meas Setup Number"(0 ("Meas Setup Number")) -> ()
        n655 = call "Bring_to_front.vi"("path"=w1340) -> ()
        n656 = global write "Trav_pos_global.vi" "Estimated Completion time"("") -> ()
        n657 = Build Array(u32 0) -> (w1349:u32[])
        n658 = property on="Table" class="Arr (strict)"("Index Values"=w1349) -> ()  [unwired: 2 in, 2 out]
      }
    }
    n659 = case shown="False" w8 {
      tunnel: w4 -> [_ w15]
      frame False {
      }
      frame True {
        n660 = local write "Table"(w15) -> ()
      }
    }
    "Multi Run Case" <- w10
  }
